vi "Demo_Main-Administrator-an.vi"() -> ()   [LabVIEW 2010]
uses:
  ControlCAN/ControlCAN.llb/DevType.ctl
  ControlCAN/ControlCAN.llb/CAN Channel.ctl
  ControlCAN/ControlCAN.llb/InitFlag.ctl
  ControlCAN/ControlCAN.llb/Mode.ctl
  ControlCAN/ControlCAN.llb/Fliter.ctl
  ControlCAN/ControlCAN.llb/VCI_CAN_OBJ.ctl
  ControlCAN/ControlCAN.llb/VCI_INIT_CONFIG.ctl
  ControlCAN/ControlCAN.llb/Return Val.ctl
  ControlCAN/ControlCAN.lvlib
panel:
  out "电流限制_回":dbl
  in  "电流限制_R":bool
  in  "电流限制_W":bool
  in  "电流限制":dbl
  in  "速度限制_R":bool
  in  "速度限制":dbl
  out "速度限制_回":dbl
  in  "速度限制_W":bool
  out "编码器线数_回":u16
  in  "编码器线数_R":bool
  in  "编码器线数_W":bool
  in  "编码器线数":u16
  in  "极对数_R":bool
  in  "极对数":u8
  out "极对数_回":u8
  in  "极对数_W":bool
  in  "电机自动校准":string(combo)="0"
  in  "电机校准_W":bool
  in  "对准角_R":bool
  in  "对准角":dbl format="%#.6f"
  out "对准角_回":dbl format="%#.6f"
  in  "对准角_W":bool
  in  "减速度_R":bool
  in  "减速度":dbl format="%#.6f"
  out "减速度_回":dbl format="%#.6f"
  in  "减速度_W":bool
  out "版本号":dbl format="%_3f"
  in  "看门狗周期_R":bool
  in  "看门狗周期":u16
  out "看门狗周期_回":u16
  in  "看门狗周期_W":bool
  in  "看门狗_W":bool
  in  "看门狗":string(combo)="开启"
  in  "监测周期_R":bool
  in  "监测周期":u16
  out "监测周期_回":u16
  in  "监测周期_W":bool
  out "ERRO7":bool
  out "ERRO6":bool
  out "ERRO5":bool
  out "ERRO4":bool
  out "ERRO3":bool
  out "高温":bool
  out "高压":bool
  out "低压":bool
  out "warn7":bool
  out "warn6":bool
  out "warn5":bool
  out "warn4":bool
  out "warn3":bool
  out "高温":bool
  out "warn1":bool
  out "warn0":bool
  out "温度":dbl format="%#.6f"
  out "转速":dbl(graph)
  out "CAN ID":u8 format="%x"
  out "数组":u8[](array[numeric]) format="%x"
  in  "DATA_SAVE_W":bool
  out "CI_K0_回":u16
  out "BI_K0_回":u16
  in  "CI_K0_R":bool
  in  "BI_K0_R":bool
  in  "CI_K0_W":bool
  in  "BI_K0_W":bool
  in  "C电流零偏":u16
  in  "B电流零偏":u16
  in  "AI_K0_R":bool
  in  "A电流零偏":u16
  out "AI_K0_回":u16
  in  "AI_K0_W":bool
  out "Sin":i32
  out "Cosin":i32
  in  "加速度_R":bool
  in  "加速度":dbl format="%#.6f"
  out "加速度_回":dbl format="%#.6f"
  in  "加速度_W":bool
  in  "速度环KI_R":bool
  in  "速度环KP_R":bool
  in  "速度环KI":dbl format="%#.6f"
  out "速度环KI_回":dbl format="%#.6f"
  in  "速度环KI_W":bool
  in  "速度环KP":dbl format="%#.6f"
  out "速度环KP_回":dbl format="%#.6f"
  in  "速度环KP_W":bool
  in  "电流环KI_R":bool
  in  "电流环KP_R":bool
  in  "电流环KI":dbl format="%#.6f"
  out "电流环KI_回":dbl format="%#.6f"
  in  "电流环KI_W":bool
  in  "电流环KP":dbl format="%#.6f"
  out "电流环KP_回":dbl format="%#.6f"
  in  "电流环KP_W":bool
  out "波形图表3":dbl(graph)
  out "波形图表2":dbl(graph)
  out "波形图表1":dbl(graph)
  out "sCnt":u32 caption="处理统计"
  out "模式_回":string(combo)="00"
  in  "模式_R":bool
  in  "设定电流_R":bool
  in  "设定位置_R":bool
  in  "设定速度_R":bool
  in  "存储路径":path
  in  "保存":bool
  out "保存_S":bool
  in  "模式_W":bool
  in  "模式":string(combo)="00"
  in  "设定电流":dbl format="%#.6f"
  out "设定电流_回":dbl format="%#.6f"
  in  "设定电流_W":bool
  in  "设定位置":dbl format="%#.6f"
  out "设定位置_回":dbl format="%#.6f"
  in  "设定位置_W":bool
  in  "设定速度":dbl format="%#.1f"
  out "设定速度_回":dbl format="%#.6f"
  in  "设定速度_W":bool
  in  "监测_W":bool
  in  "监测":string(combo)="30"
  out "电机ID_R":u32
  in  "Clear":bool
  out "Ualfa":dbl format="%#.6f"
  out "Ubate":dbl format="%#.6f"
  out "Uq":dbl format="%#.6f"
  out "Ud":dbl format="%#.6f"
  out "PWM1":u16
  out "PWM2":u16
  out "PWM3":u16
  out "sector":u8
  out "Iqnow":dbl
  out "Idnow":dbl
  out "Ialfa":dbl
  out "Ibeta":dbl
  out "A电流":dbl
  out "C电流":dbl
  out "B电流":dbl
  out "供电电压":dbl
  out "机械角度":dbl format="%.2f"
  out "电气角度":dbl
  out "转速":dbl
  out "CAN STD_ID":u32 format="%x"
  in  "电机ID":string(combo)="00"
  in  "电机ID_W":bool
  out "RecvCnt":u32 caption="接收统计"
  out "SendCnt":u32 caption="发送统计"
  in  "Format":u8(ring) items=["标准帧", "扩展帧"]
  in  "Type":u8(ring) items=["数据帧", "远程帧"]
  in  "Data":string="00 01 02 03 04 05 06 07"
  in  "ID":u32=291 format="0x%x"
  in  "Send":bool
  in  "RcvEnable":bool=TRUE
  out "Open":bool
  in  "Fliter":T1=1 items=["接收所有类型"=1, "只接收标准帧"=2, "只接收扩展帧"=3]
  in  "kBaudRate":u8(ring)=12 caption="波特率" items=["5k bps"=1, "10k bps"=2, "20k bps"=3, "40k bps"=4, "50k bps"=5, "80k bps"=6, "100k bps"=7, "125k bps"=8, "200k bps"=9, "250k bps"=10, "400k bps"=11, "500k bps"=12, "666k bps"=13, "800k bps"=14, "1000k bps"=15, "33.33k bps"=16, "66.66k bps"=17, "83.33k bps"=18]
  in  "Mode":T2 caption="工作模式" items=["正常工作", "仅侦听模式", "自测模式（环回）"]
  in  "InitFlag":T3 caption="初始化参数" items=["使用Flash参数", "使用界面设置参数"]
  in  "AccMask":u32=4294967295 caption="接收屏蔽码" format="%08x"
  in  "AccCode":u32 caption="接收过滤码" format="%08x"
  in  "Close":bool
  in  "Open":bool
  in  "Channel":T4 caption="CAN通道" items=["通道1", "通道2"]
  in  "DevType":T5=3 caption="设备类型" items=["USB-CAN"=2, "USB-CAN2"=3]
  # "发送指令帧包"
  # "CAN\n  ID"
  # "DATA"
  # "DATA"
  # "DATA"
  # "0"
  # "1"
  # "7"
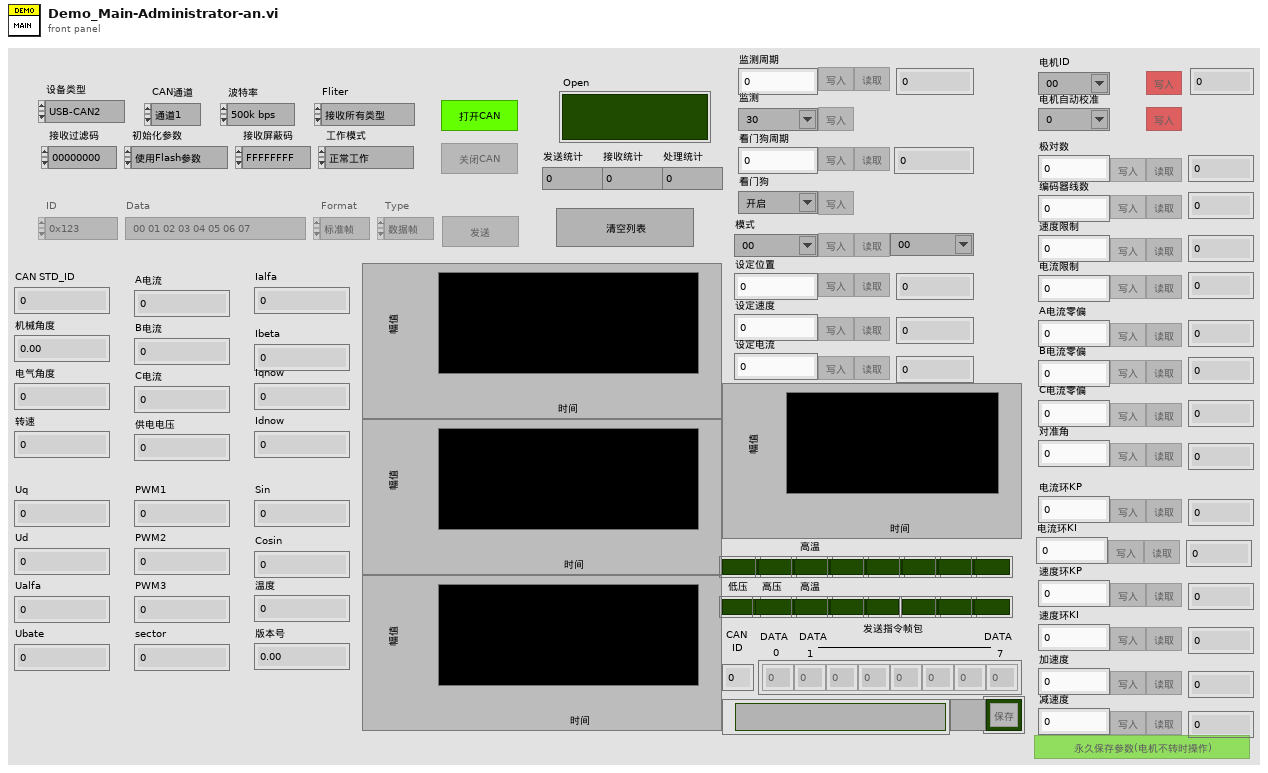
[diagram p1: front panel]
types:
  T1 = typedef "ControlCAN.lvlib/Fliter.ctl" = u8
  T2 = typedef "ControlCAN.lvlib/Mode.ctl" = u8
  T3 = typedef "ControlCAN.lvlib/InitFlag.ctl" = u32
  T4 = typedef "ControlCAN.lvlib/CAN Channel.ctl" = u32
  T5 = typedef "ControlCAN.lvlib/DevType.ctl" = u32
  T6 = typedef "ControlCAN.lvlib/VCI_CAN_OBJ.ctl" = cluster{"ID":u32, "TimeStamp":u32, "TimeFlag":u8, "SendType":u8, "RemoteFlag":u8, "ExternFlag":u8, "DataLen":u8, "Data":u8[], "Reserved":u8[]}
  T7 = cluster{"Type":enum16{"接收", "发送"}, "Channel":T4, "Time":timestamp, "VCI_CAN_OBJ":T6}[]
  T8 = typedef "ControlCAN.lvlib/VCI_INIT_CONFIG.ctl" = cluster{"AccCode":u32, "AccMask":u32, "InitFlag":T3, "Fliter":T1, "Timing0":u8, "Timing1":u8, "Mode":T2}
  T9 = cluster{"DevType":T5, "DevIndex":u32, "CanIndex":T4, "VCI_INIT_CONFIG":T8}
  T10 = typedef "ControlCAN.lvlib/Return Val.ctl" = i32
  T11 = enum16{"open", "replace", "create", "open or create", "replace or create", "replace or create with confirmation"}
  T12 = cluster{"[0]":cluster{"Type":enum16{"接收", "发送"}, "Channel":T4, "Time":timestamp, "VCI_CAN_OBJ":T6}}
  T13 = cluster{"Type":enum16{"接收", "发送"}, "Channel":T4, "Time":timestamp, "VCI_CAN_OBJ":T6}
  T14 = cluster{"Data[0]":u8, "Data[1]":u8, "Data[2]":u8, "Data[3]":u8, "Data[4]":u8, "Data[5]":u8, "Data[6]":u8, "Data[7]":u8}
  T15 = cluster{"Boolean array[0]":bool, "Boolean array[1]":bool, "Boolean array[2]":bool, "Boolean array[3]":bool, "Boolean array[4]":bool, "Boolean array[5]":bool, "Boolean array[6]":bool, "Boolean array[7]":bool}
  T16 = enum32{"invalid app kind", "Development System", "Run Time System", "Student Edition", "Embedded LabVIEW", "Evaluation", "Custom"}
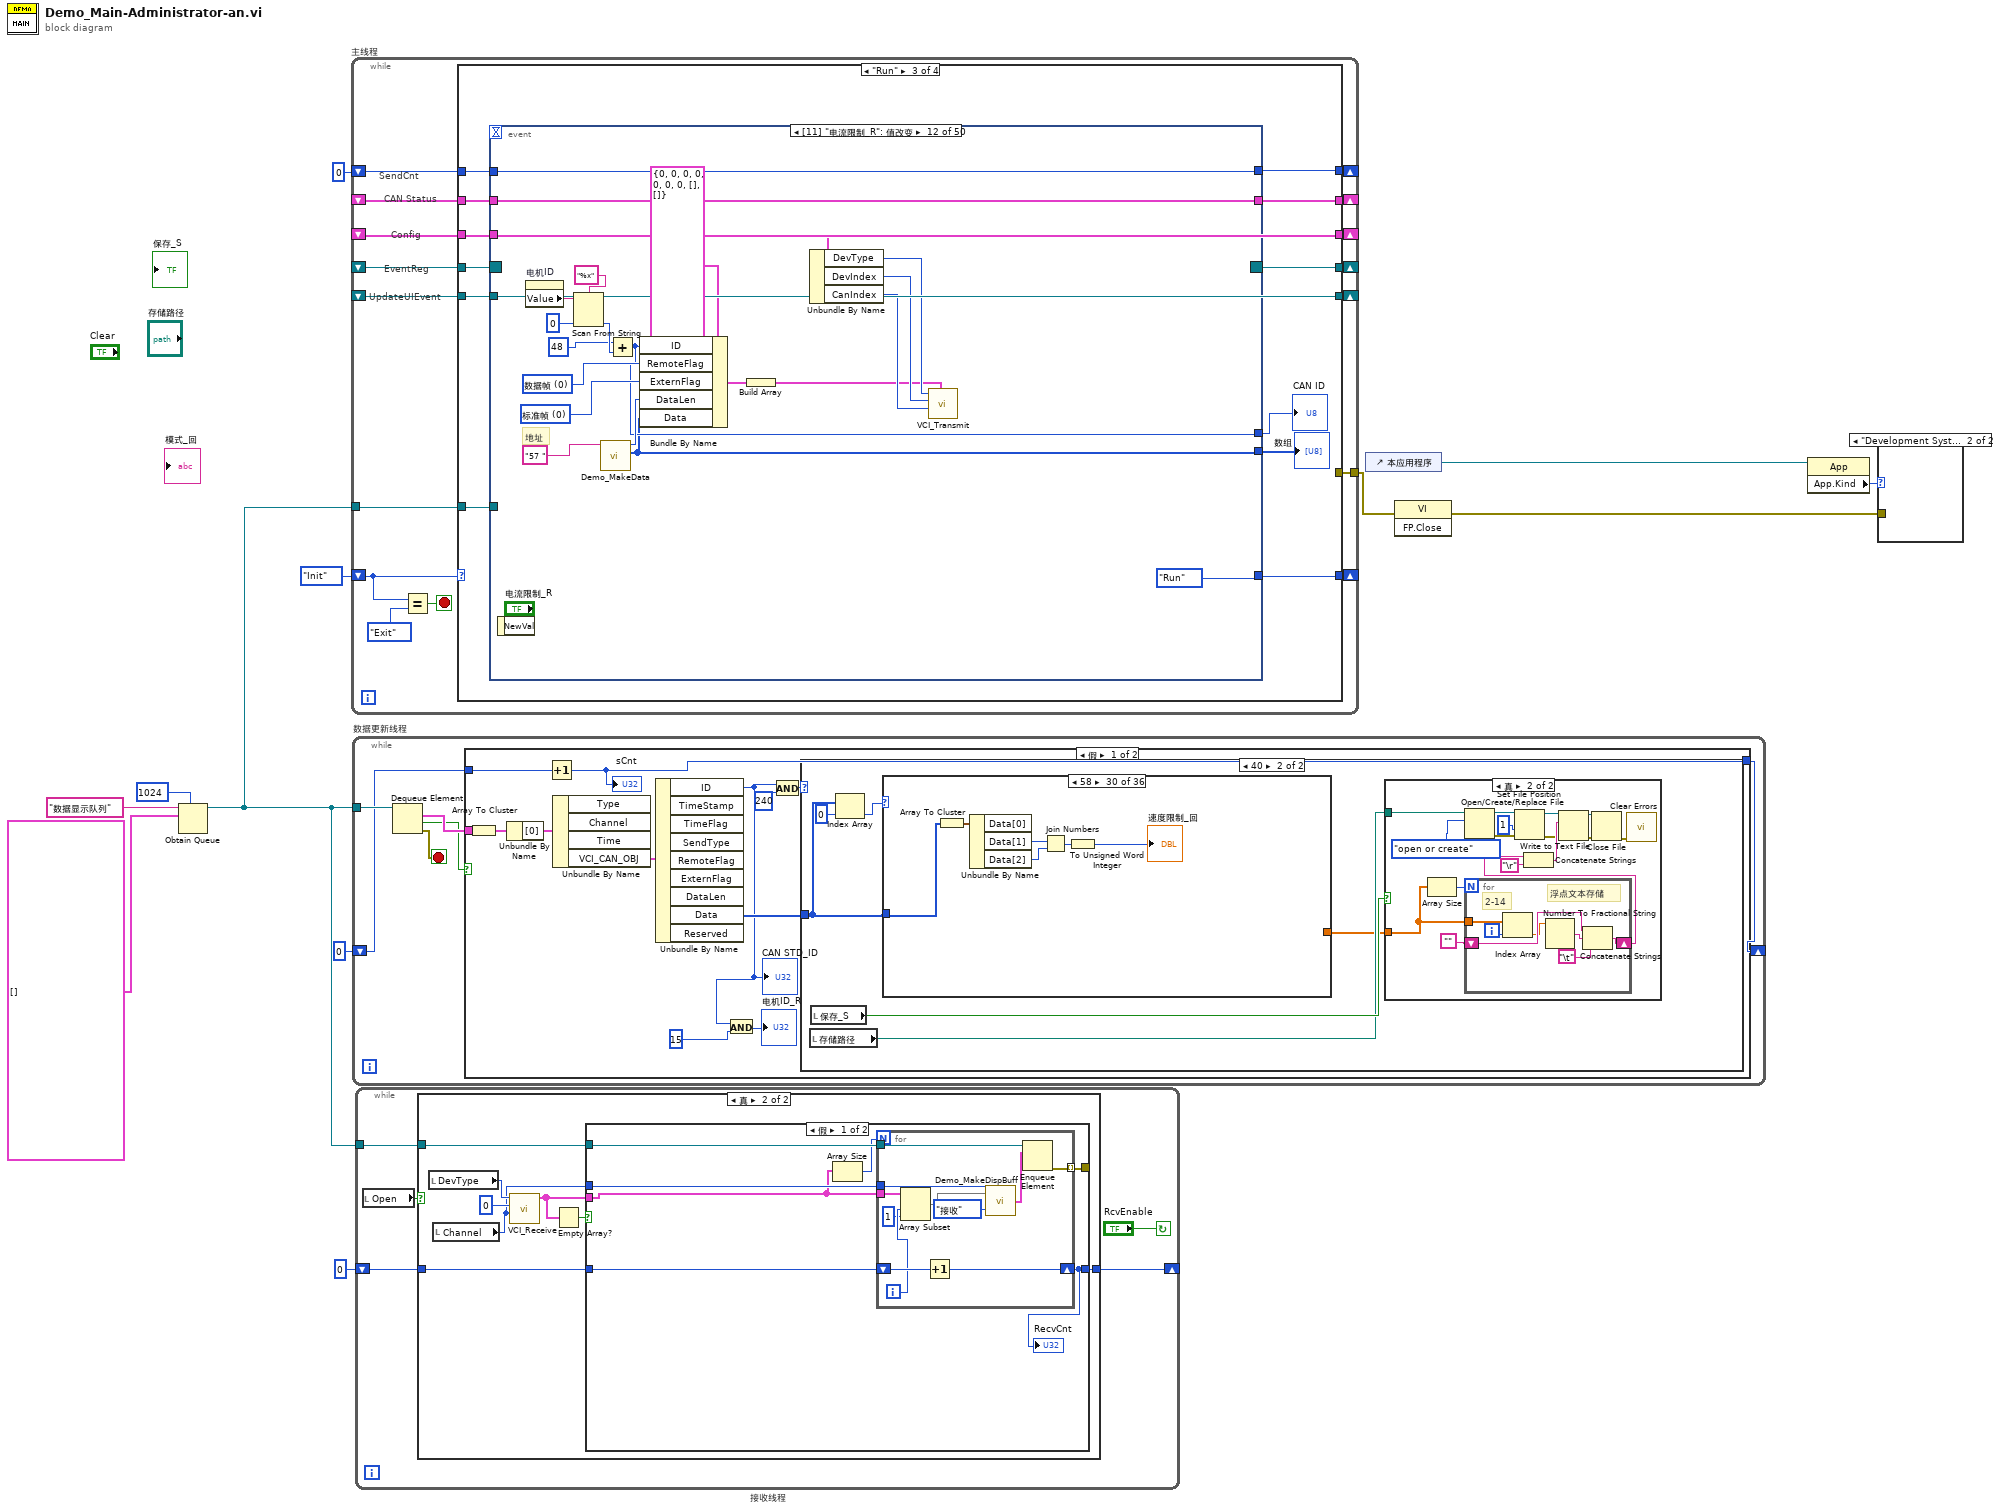
[diagram p0: block diagram]
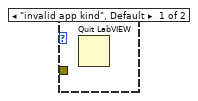
[diagram p2: hidden frame]
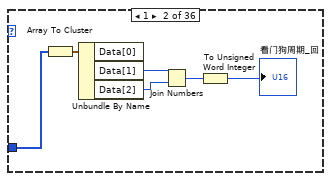
[diagram p6: hidden frame]
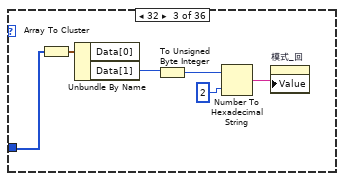
[diagram p7: hidden frame]
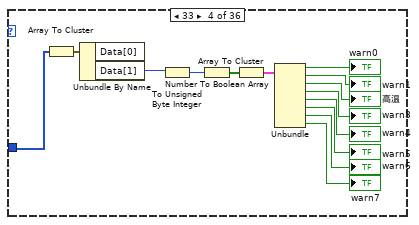
[diagram p8: hidden frame]
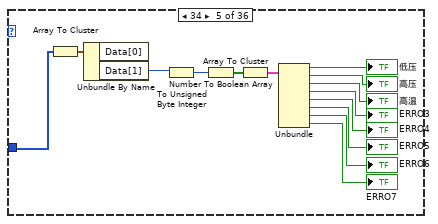
[diagram p9: hidden frame]
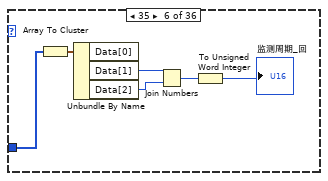
[diagram p10: hidden frame]
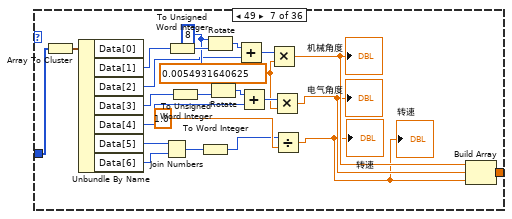
[diagram p11: hidden frame]
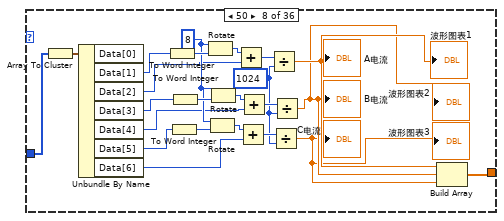
[diagram p12: hidden frame]
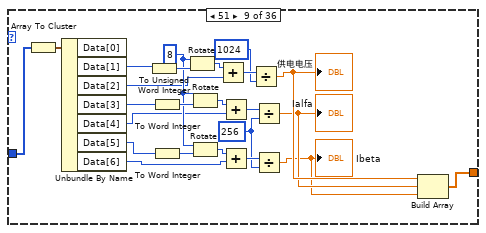
[diagram p13: hidden frame]
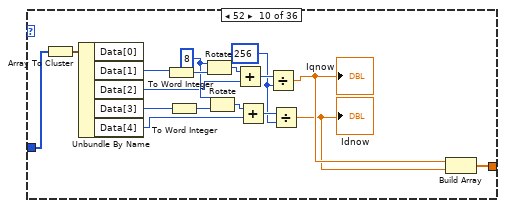
[diagram p14: hidden frame]
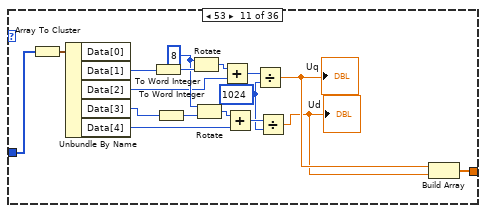
[diagram p15: hidden frame]
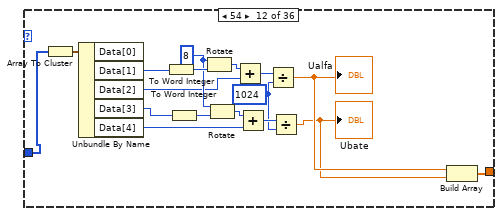
[diagram p16: hidden frame]
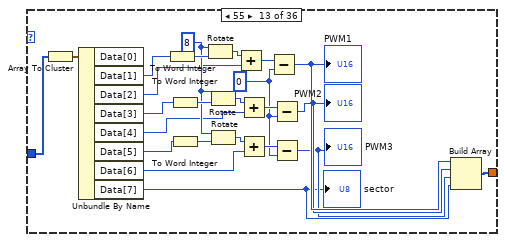
[diagram p17: hidden frame]
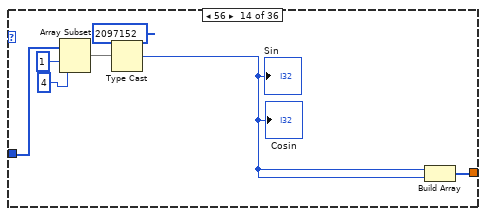
[diagram p18: hidden frame]
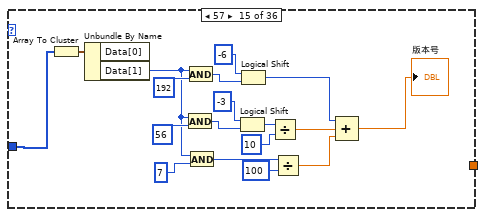
[diagram p19: hidden frame]
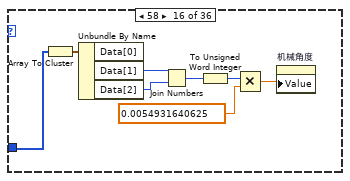
[diagram p20: hidden frame]
diagram:
  n1 = Obtain Queue(max queue size (-1, unlimited)=1024, name (unnamed)="数据显示队列" ("名称（未命名）"), element data type=T7 []) -> (queue out=w9:refnum<queue>)  [unwired: 2 in, 2 out]
  n2 = while "主线程" {
    shift-right: [w24] -> _
    shift-left: enum16{"Init", "Wait", "Run", "Exit"}."Init" -> [w27]
    shift-right: [w25] -> _
    shift-left: _ -> [w26]
    shift-right: [w23] -> _
    shift-left: _ -> [w22]
    tunnel: w9 -> [w21]
    shift-right: [w19] -> _
    shift-left: _ -> [w18]
    shift-right: [w17] -> _
    shift-left: _ -> [w16]
    shift-right: [w14] -> _
    shift-left: u32 0 -> [w15]
    tunnel: [w13] -> w4
    stop <- w28 stop-if-true
    # "CAN Status"
    # "Config"
    # "EventReg"
    # "UpdateUIEvent"
    # "SendCnt"
    n3 = Equal?(x=w27, y=enum16{"Init", "Wait", "Run", "Exit"}."Exit") -> (x = y?=w28:bool)
    n4 = case shown="\"Run\"" w27 {
      tunnel: w26 -> [_ w57 w158 w1270]
      tunnel: [w48 w56 w157 w1270] -> w25
      tunnel: [enum16{"Init", "Wait", "Run", "Exit"}."Wait" w53 w160 enum16{"Init", "Wait", "Run", "Exit"}."Exit"] -> w24
      tunnel: [w44 w54 w156 w1268] -> w23
      tunnel: w22 -> [_ w55 w156 w1268]
      tunnel: w21 -> [_ w52 w159 w1274]
      tunnel: [w36 w51 w154 w1273] -> w19
      tunnel: w18 -> [_ w51 w155 w1273]
      tunnel: [w35 w50 w153 w1271] -> w17
      tunnel: w16 -> [_ w50 w153 w1271]
      tunnel: w15 -> [w33 w49 w152 w1266]
      tunnel: [w33 w49 w151 w1266] -> w14
      tunnel: [_ _ _ errorcluster {"status"=FALSE, "code"=0, "source"=""} ("error constant")] -> w13
      frame "Init", Default {
        w37 = cluster{"CANOpen":bool} {"CANOpen"=FALSE}  # UpdateUI
        w47 = T9 {"DevType"=2, "DevIndex"=0, "CanIndex"=0, "VCI_INIT_CONFIG"={"AccCode"=0, "AccMask"=0, "InitFlag"=0, "Fliter"=0, "Timing0"=0, "Timing1"=0, "Mode"=0}}  # Config
        w48 = cluster{"Open":bool, "SendCnt":u32} {"Open"=FALSE, "SendCnt"=0}  # CAN Status
        n5 = property class="VI"("Front Panel.Closeable"=TRUE ("前面板窗口:可关闭")) -> ()  [unwired: 2 in, 2 out]
        n6 = invoke class="VI" method="Default Vals.Reinit All"() -> ()  [unwired: 3 in, 3 out]
        n7 = call "Demo_GetT0T1.vi"("kBaudRate"="kBaudRate") -> ("Timing0"=w30:u8, "Timing1"=w29:u8)
        n8 = Bundle By Name(cluster=w47, "DevType"="DevType", "CanIndex"="Channel", "VCI_INIT_CONFIG.AccCode"="AccCode", "VCI_INIT_CONFIG.AccMask"="AccMask", "VCI_INIT_CONFIG.InitFlag"="InitFlag", "VCI_INIT_CONFIG.Fliter"="Fliter", "VCI_INIT_CONFIG.Timing0"=w30, "VCI_INIT_CONFIG.Timing1"=w29, "VCI_INIT_CONFIG.Mode"="Mode") -> (w44:T9)
        n9 = local write "RcvEnable"(TRUE ("RcvEnable")) -> ()
        n10 = Create User Event(user event datatype=w37) -> (user event=w35:refnum<user-event>)  [unwired: 1 in, 1 out]
        n11 = register-events(w35) -> (reference out=w36:refnum<event-registration>)  [unwired: 2 in, 1 out]
      }
      frame "Wait" {
        n12 = event shown="[1] 前面板关闭？" {
          selector: _ -> [_ _ _ _ _ _ _ _ _ _]
          dyn-events: _ -> [_ _ _ _ _ _ _ _ _ _]
          timeout: _ -> [_ _ _ _ _ _ _ _ _ _]
          tunnel: w57 -> [w61 w101 w111 w116 w121 w126 w131 w136 w143 w148]
          tunnel: [w60 w101 w111 w116 w121 w126 w131 w136 w143 w148] -> w56
          tunnel: w55 -> [w71 w100 w110 w115 w120 w125 w130 w135 w142 w147]
          tunnel: [w71 w100 w109 w113 w118 w123 w128 w133 w141 w145] -> w54
          tunnel: [w62 enum16{"Init", "Wait", "Run", "Exit"}."Exit" enum16{"Init", "Wait", "Run", "Exit"}."Wait" enum16{"Init", "Wait", "Run", "Exit"}."Wait" enum16{"Init", "Wait", "Run", "Exit"}."Wait" enum16{"Init", "Wait", "Run", "Exit"}."Wait" enum16{"Init", "Wait", "Run", "Exit"}."Wait" enum16{"Init", "Wait", "Run", "Exit"}."Wait" enum16{"Init", "Wait", "Run", "Exit"}."Wait" enum16{"Init", "Wait", "Run", "Exit"}."Wait"] -> w53
          tunnel: w52 -> [_ _ _ _ _ _ _ _ _ _]
          tunnel: w50 -> [w59 _ _ _ _ _ _ _ _ _]
          event "Open": Value Change {
            w65 = T10 1 items=["OK"=1, "ERROR1"=0, "ERROR2"=-1] ("y")
            # "打开CAN的步骤：\n1.Open\n2.Init\n3.Start"
            n13 = event-data() -> ()  [unwired: 2 out]
            n14 = Unbundle By Name(w71) -> ("DevType"=w70:T5, "DevIndex"=w69:u32)
            n15 = call "VCI_OpenDevice.vi"("DevIndex"=w69, "DevType"=w70) -> ("error out"=w66:errorcluster, "Return Val"=w68:T10)  [unwired: 2 in, 6 out]
            n16 = Equal?(x=w68, y=w65) -> (x = y?=w67:bool)
            n17 = case shown="真" w67 {
              tunnel: w66 -> [_ w86]
              tunnel: w71 -> [_ w85]
              tunnel: w65 -> [_ w77]
              tunnel: [_ w76] -> w58
              frame False {
              }
              frame True {
                n18 = Unbundle By Name(w85) -> ("VCI_INIT_CONFIG"=w84:T8, "DevType"=w80:T5, "DevIndex"=w79:u32, "CanIndex"=w78:T4)
                n19 = call "VCI_InitCAN.vi"("VCI_INIT_CONFIG"=w84, "error in (no error)"=w86, "CANIndex"=w78, "DevIndex"=w79, "DevType"=w80) -> ("error out"=w81:errorcluster, "Return Val"=w83:T10)  [unwired: 5 out]
                n20 = Equal?(x=w77, y=w83) -> (x = y?=w82:bool)
                n21 = case shown="真" w82 {
                  tunnel: w81 -> [_ w97]
                  tunnel: w80 -> [_ w96]
                  tunnel: w79 -> [_ w95]
                  tunnel: w78 -> [_ w94]
                  tunnel: w77 -> [_ w92]
                  tunnel: [_ w88] -> w76
                  frame False {
                  }
                  frame True {
                    n22 = call "VCI_StartCAN.vi"("error in (no error)"=w97, "CANIndex"=w94, "DevIndex"=w95, "DevType"=w96) -> ("error out"=w90:errorcluster, "Return Val"=w93:T10)  [unwired: 6 out]
                    n23 = Unbundle By Name(w90) -> ("status"=w87:bool)
                    n24 = Equal?(x=w92, y=w93) -> (x = y?=w91:bool)
                    n25 = Not(x=w87) -> (.not. x?=w89:bool)
                    n26 = And(x=w91, y=w89) -> (x .and. y?=w88:bool)
                  }
                }
              }
            }
            n27 = case shown="真" w58 {
              tunnel: w59 -> [_ w75]
              tunnel: w58 -> [_ w73]
              frame False {
              }
              frame True {
                n28 = Bundle By Name(cluster=cluster{"CANOpen":bool} {"CANOpen"=FALSE} ("事件数据"), "CANOpen"=w73) -> (w72:cluster{"CANOpen":bool})
                n29 = Generate User Event(user event=w75, event data cluster=w72) -> ()  [unwired: 1 in, 2 out]
              }
            }
            n30 = Select(t=enum16{"Init", "Wait", "Run", "Exit"}."Run", s=w58, f=enum16{"Init", "Wait", "Run", "Exit"}."Wait") -> (s? t:f=w62:enum16{"Init", "Wait", "Run", "Exit"})
            n31 = Bundle By Name(cluster=w61, "Open"=w58) -> (w60:cluster{"Open":bool, "SendCnt":u32})
          }
          event Panel Close? {
            n32 = event-data() -> ()  [unwired: 2 out]
            n33 = event-data("Discard?"=TRUE ("放弃？")) -> ()  [unwired: 1 in, 1 out]
          }
          event Value Change {
            w107 = T5 3 items=["USB-CAN"=2, "USB-CAN2"=3] ("y")
            n34 = event-data() -> ("NewVal"=w108:T5)  [unwired: 1 out]
            n35 = Equal?(x=w108, y=w107) -> (x = y?=w106:bool)
            n36 = Bundle By Name(cluster=w110, "DevType"=w108) -> (w109:T9)
            n37 = Select(t=i32[] [] ("禁用项[]"), s=w106, f=i32[] [1] ("禁用项[]")) -> (s? t:f=w105:i32[])
            n38 = property on="Channel" class="Ring (严格)"("Disabled Items []"=w105) -> ()  [unwired: 2 in, 2 out]
          }
          event Value Change {
            n39 = event-data() -> ("NewVal"=w114:T4)  [unwired: 1 out]
            n40 = Bundle By Name(cluster=w115, "CanIndex"=w114) -> (w113:T9)
          }
          event "AccCode": Value Change {
            n41 = event-data() -> ("NewVal"=w119:u32)  [unwired: 1 out]
            n42 = Bundle By Name(cluster=w120, "VCI_INIT_CONFIG.AccCode"=w119) -> (w118:T9)
          }
          event "AccMask": Value Change {
            n43 = event-data() -> ("NewVal"=w124:u32)  [unwired: 1 out]
            n44 = Bundle By Name(cluster=w125, "VCI_INIT_CONFIG.AccMask"=w124) -> (w123:T9)
          }
          event Value Change {
            n45 = event-data() -> ("NewVal"=w129:T3)  [unwired: 1 out]
            n46 = Bundle By Name(cluster=w130, "VCI_INIT_CONFIG.InitFlag"=w129) -> (w128:T9)
          }
          event Value Change {
            n47 = event-data() -> ("NewVal"=w134:T2)  [unwired: 1 out]
            n48 = Bundle By Name(cluster=w135, "VCI_INIT_CONFIG.Mode"=w134) -> (w133:T9)
          }
          event "kBaudRate": Value Change {
            n49 = event-data() -> ("NewVal"=w139:u8)  [unwired: 1 out]
            n50 = call "Demo_GetT0T1.vi"("kBaudRate"=w139) -> ("Timing0"=w138:u8, "Timing1"=w137:u8)
            n51 = Bundle By Name(cluster=w142, "VCI_INIT_CONFIG.Timing0"=w138, "VCI_INIT_CONFIG.Timing1"=w137) -> (w141:T9)
          }
          event Value Change {
            n52 = event-data() -> ("NewVal"=w146:T1)  [unwired: 1 out]
            n53 = Bundle By Name(cluster=w147, "VCI_INIT_CONFIG.Fliter"=w146) -> (w145:T9)
          }
        }
      }
      frame "Run" {
        n54 = event shown="[11] \"电流限制_R\": 值改变" {
          selector: w155 -> [_ _ _ _ _ _ _ _ _ _ _ _ _ _ _ _ _ _ _ _ _ _ _ _ _ _ _ _ _ _ _ _ _ _ _ _ _ _ _ _ _ _ _ _ _ _ _ _ _ _]
          dyn-events: [_ _ _ _ _ _ _ _ _ _ _ _ _ _ _ _ _ _ _ _ _ _ _ _ _ _ _ _ _ _ _ _ _ _ _ _ _ _ _ _ _ _ _ _ _ _ _ _ _ _] -> w154
          timeout: _ -> [_ _ _ _ _ _ _ _ _ _ _ _ _ _ _ _ _ _ _ _ _ _ _ _ _ _ _ _ _ _ _ _ _ _ _ _ _ _ _ _ _ _ _ _ _ _ _ _ _ _]
          tunnel: [enum16{"Init", "Wait", "Run", "Exit"}."Run" enum16{"Init", "Wait", "Run", "Exit"}."Run" enum16{"Init", "Wait", "Run", "Exit"}."Run" enum16{"Init", "Wait", "Run", "Exit"}."Run" enum16{"Init", "Wait", "Run", "Exit"}."Run" enum16{"Init", "Wait", "Run", "Exit"}."Run" enum16{"Init", "Wait", "Run", "Exit"}."Run" enum16{"Init", "Wait", "Run", "Exit"}."Run" enum16{"Init", "Wait", "Run", "Exit"}."Run" enum16{"Init", "Wait", "Run", "Exit"}."Run" enum16{"Init", "Wait", "Run", "Exit"}."Run" enum16{"Init", "Wait", "Run", "Exit"}."Run" enum16{"Init", "Wait", "Run", "Exit"}."Run" enum16{"Init", "Wait", "Run", "Exit"}."Run" enum16{"Init", "Wait", "Run", "Exit"}."Run" enum16{"Init", "Wait", "Run", "Exit"}."Run" enum16{"Init", "Wait", "Run", "Exit"}."Run" enum16{"Init", "Wait", "Run", "Exit"}."Run" enum16{"Init", "Wait", "Run", "Exit"}."Run" enum16{"Init", "Wait", "Run", "Exit"}."Run" enum16{"Init", "Wait", "Run", "Exit"}."Run" enum16{"Init", "Wait", "Run", "Exit"}."Run" enum16{"Init", "Wait", "Run", "Exit"}."Run" enum16{"Init", "Wait", "Run", "Exit"}."Run" enum16{"Init", "Wait", "Run", "Exit"}."Run" enum16{"Init", "Wait", "Run", "Exit"}."Run" enum16{"Init", "Wait", "Run", "Exit"}."Run" enum16{"Init", "Wait", "Run", "Exit"}."Run" enum16{"Init", "Wait", "Run", "Exit"}."Run" enum16{"Init", "Wait", "Run", "Exit"}."Run" enum16{"Init", "Wait", "Run", "Exit"}."Run" enum16{"Init", "Wait", "Run", "Exit"}."Run" enum16{"Init", "Wait", "Run", "Exit"}."Run" enum16{"Init", "Wait", "Run", "Exit"}."Run" enum16{"Init", "Wait", "Run", "Exit"}."Run" enum16{"Init", "Wait", "Run", "Exit"}."Run" enum16{"Init", "Wait", "Run", "Exit"}."Run" enum16{"Init", "Wait", "Run", "Exit"}."Run" enum16{"Init", "Wait", "Run", "Exit"}."Run" enum16{"Init", "Wait", "Run", "Exit"}."Run" enum16{"Init", "Wait", "Run", "Exit"}."Run" enum16{"Init", "Wait", "Run", "Exit"}."Run" enum16{"Init", "Wait", "Run", "Exit"}."Run" enum16{"Init", "Wait", "Run", "Exit"}."Run" enum16{"Init", "Wait", "Run", "Exit"}."Run" enum16{"Init", "Wait", "Run", "Exit"}."Run" enum16{"Init", "Wait", "Run", "Exit"}."Run" enum16{"Init", "Wait", "Run", "Exit"}."Run" enum16{"Init", "Wait", "Run", "Exit"}."Run" w1259] -> w160
          tunnel: w159 -> [_ _ _ _ _ _ _ _ _ _ _ _ _ _ _ _ _ _ _ _ _ _ _ _ _ _ _ _ _ _ _ _ _ _ _ _ _ _ _ _ _ _ _ _ _ _ _ _ _ _]
          tunnel: [w162 w179 w196 w219 w241 w262 w286 w307 w334 w355 w382 w403 w427 w448 w469 w488 w509 w525 w563 w584 w610 w636 w662 w688 w714 w740 w766 w792 w818 w842 w866 w890 w917 w938 w959 w980 w1001 w1022 w1043 w1064 w1085 w1106 w1127 w1148 w1169 w1190 w1211 w1239 w1245 w1264] -> w157
          tunnel: w158 -> [w162 w179 w196 w219 w241 w262 w286 w307 w334 w355 w382 w403 w427 w448 w469 w488 w509 w525 w563 w584 w610 w636 w662 w688 w714 w740 w766 w792 w818 w842 w866 w890 w917 w938 w959 w980 w1001 w1022 w1043 w1064 w1085 w1106 w1127 w1148 w1169 w1190 w1211 w1239 w1247 w1264]
          tunnel: w156 -> [_ w174 w186 w201 w224 w245 w267 w290 w315 w338 w360 w386 w408 w431 w458 w474 w492 w515 w545 w567 w595 w618 w644 w667 w693 w719 w745 w771 w797 w823 w847 w871 w898 w921 w942 w963 w984 w1005 w1026 w1047 w1068 w1089 w1110 w1131 w1152 w1173 w1194 _ w1252 _]
          tunnel: w153 -> [_ _ _ _ _ _ _ _ _ _ _ _ _ _ _ _ _ _ _ _ _ _ _ _ _ _ _ _ _ _ _ _ _ _ _ _ _ _ _ _ _ _ _ _ _ _ _ _ w1244 _]
          tunnel: w152 -> [w161 w167 w195 w218 w240 w261 w285 w306 w333 w354 w381 w402 w426 w447 w468 w487 w508 w524 w562 w583 w609 w635 w661 w687 w713 w739 w765 w791 w817 w841 w865 w889 w916 w937 w958 w979 w1000 w1021 w1042 w1063 w1084 w1105 w1126 w1147 w1168 w1189 w1210 w1238 w1240 w1258]
          tunnel: [w161 w166 w195 w218 w240 w261 w285 w306 w333 w354 w381 w402 w426 w447 w468 w487 w508 w524 w562 w583 w609 w635 w661 w687 w713 w739 w765 w791 w817 w841 w865 w889 w916 w937 w958 w979 w1000 w1021 w1042 w1063 w1084 w1105 w1126 w1147 w1168 w1189 w1210 w1238 w1240 w1258] -> w151
          tunnel: [_ _ w182 w199 w222 w243 w264 w288 w313 w336 w358 w384 w406 w429 w450 w472 w490 w511 w543 w565 w586 w612 w638 w664 w690 w716 w742 w768 w795 w820 w844 w868 w896 w919 w940 w961 w982 w1003 w1024 w1045 w1066 w1087 w1108 w1129 w1150 w1171 w1192 _ _ _] -> w150
          tunnel: [_ _ w181 w200 w223 w244 w265 w289 w314 w337 w359 w385 w407 w430 w449 w473 w491 w514 w542 w564 w585 w611 w637 w663 w689 w715 w741 w767 w794 w819 w843 w867 w897 w918 w939 w960 w981 w1002 w1023 w1044 w1065 w1086 w1109 w1128 w1149 w1170 w1193 _ _ _] -> w149
          event Timeout {
            n55 = event-data() -> ()  [unwired: 3 out]
          }
          event "Send": Value Change {
            n56 = event-data() -> ()  [unwired: 2 out]
            n57 = Increment(x=w167) -> (x+1=w166:u32)
            "SendCnt" <- w166
            n58 = call "Demo_MakeData.vi"("DataString"="Data") -> ("Data"=w169:u8[], "DataLen"=w170:u8)  [unwired: 9 out]
            n59 = Bundle By Name(cluster=T6 {"ID"=0, "TimeStamp"=0, "TimeFlag"=0, "SendType"=0, "RemoteFlag"=0, "ExternFlag"=0, "DataLen"=0, "Data"=[], "Reserved"=[]} ("Send"), "ID"="ID", "RemoteFlag"="Type", "ExternFlag"="Format", "DataLen"=w170, "Data"=w169) -> (w164:T6)
            n60 = Build Array(w164) -> (w165:T6[])
            n61 = Unbundle By Name(w174) -> ("DevType"=w173:T5, "DevIndex"=w172:u32, "CanIndex"=w168:T4)
            n62 = call "VCI_Transmit.vi"("Buffer"=w165, "CANIndex"=w168, "DevIndex"=w172, "DevType"=w173) -> ()  [unwired: 1 in, 7 out]
          }
          event "电机ID_W": Value Change {
            w185 = u8 0 items=["数据帧", "遥控帧"]
            w181 = u32 138
            w184 = u8 0 items=["标准帧", "扩展帧"]
            n63 = event-data() -> ()  [unwired: 2 out]
            n64 = call "Demo_MakeData.vi"("DataString"="电机ID") -> ("Data"=w182:u8[], "DataLen"=w190:u8)  [unwired: 9 out]
            n65 = Bundle By Name(cluster=T6 {"ID"=0, "TimeStamp"=0, "TimeFlag"=0, "SendType"=0, "RemoteFlag"=0, "ExternFlag"=0, "DataLen"=0, "Data"=[], "Reserved"=[]} ("Send"), "ID"=w181, "RemoteFlag"=w185, "ExternFlag"=w184, "DataLen"=w190, "Data"=w182) -> (w187:T6)
            n66 = Build Array(w187) -> (w188:T6[])
            n67 = Unbundle By Name(w186) -> ("DevType"=w192:T5, "DevIndex"=w191:u32, "CanIndex"=w189:T4)
            n68 = call "VCI_Transmit.vi"("Buffer"=w188, "CANIndex"=w189, "DevIndex"=w191, "DevType"=w192) -> ()  [unwired: 1 in, 7 out]
          }
          event "电机校准_W": Value Change {
            w216 = u8 0 items=["数据帧", "遥控帧"]
            w217 = u8 0 items=["标准帧", "扩展帧"]
            # "地址"
            n69 = event-data() -> ()  [unwired: 2 out]
            n70 = property on="电机ID" class="CmbBox"() -> ("Value"=w207:string)  [unwired: 2 in, 2 out]
            n71 = Concatenate Strings("20 ", "AA 01 02 03 04 05 55") -> (w203:string)
            n72 = Scan From String(format string="%x" ("格式字符串"), input string=w207, default 1=u8 0) -> (output 1=w204:u8)  [unwired: 2 in, 3 out]
            n73 = call "Demo_MakeData.vi"("DataString"=w203) -> ("Data"=w199:u8[], "DataLen"=w212:u8)  [unwired: 9 out]
            n74 = Add(x=u32 16, y=w204) -> (x+y=w200:u32)
            n75 = Bundle By Name(cluster=T6 {"ID"=0, "TimeStamp"=0, "TimeFlag"=0, "SendType"=0, "RemoteFlag"=0, "ExternFlag"=0, "DataLen"=0, "Data"=[], "Reserved"=[]} ("Send"), "ID"=w200, "RemoteFlag"=w216, "ExternFlag"=w217, "DataLen"=w212, "Data"=w199) -> (w215:T6)
            n76 = Build Array(w215) -> (w214:T6[])
            n77 = Unbundle By Name(w201) -> ("DevType"=w210:T5, "DevIndex"=w211:u32, "CanIndex"=w213:T4)
            n78 = call "VCI_Transmit.vi"("Buffer"=w214, "CANIndex"=w213, "DevIndex"=w211, "DevType"=w210) -> ()  [unwired: 1 in, 7 out]
          }
          event "极对数_W": Value Change {
            w236 = u8 0 items=["数据帧", "遥控帧"]
            w237 = u8 0 items=["标准帧", "扩展帧"]
            # "索引地址"
            n79 = event-data() -> ()  [unwired: 2 out]
            n80 = property on="电机ID" class="CmbBox"() -> ("Value"=w228:string)  [unwired: 2 in, 2 out]
            n81 = Scan From String(format string="%x" ("格式字符串"), input string=w228, default 1=u8 0) -> (output 1=w225:u8)  [unwired: 2 in, 3 out]
            n82 = Add(x=u32 16, y=w225) -> (x+y=w223:u32)
            n83 = Build Array(u8 94, "极对数") -> (w222:u8[])
            n84 = Bundle By Name(cluster=T6 {"ID"=0, "TimeStamp"=0, "TimeFlag"=0, "SendType"=0, "RemoteFlag"=0, "ExternFlag"=0, "DataLen"=0, "Data"=[], "Reserved"=[]} ("Send"), "ID"=w223, "RemoteFlag"=w236, "ExternFlag"=w237, "DataLen"=u8 2, "Data"=w222) -> (w235:T6)
            n85 = Build Array(w235) -> (w234:T6[])
            n86 = Unbundle By Name(w224) -> ("DevType"=w231:T5, "DevIndex"=w232:u32, "CanIndex"=w233:T4)
            n87 = call "VCI_Transmit.vi"("Buffer"=w234, "CANIndex"=w233, "DevIndex"=w232, "DevType"=w231) -> ()  [unwired: 1 in, 7 out]
          }
          event "极对数_R": Value Change {
            w248 = u8 0 items=["数据帧", "遥控帧"]
            w247 = u8 0 items=["标准帧", "扩展帧"]
            # "地址"
            n88 = event-data() -> ()  [unwired: 2 out]
            n89 = property on="电机ID" class="CmbBox"() -> ("Value"=w257:string)  [unwired: 2 in, 2 out]
            n90 = Scan From String(format string="%x" ("格式字符串"), input string=w257, default 1=u8 0) -> (output 1=w260:u8)  [unwired: 2 in, 3 out]
            n91 = call "Demo_MakeData.vi"("DataString"="5E") -> ("Data"=w243:u8[], "DataLen"=w252:u8)  [unwired: 9 out]
            n92 = Add(x=u32 48, y=w260) -> (x+y=w244:u32)
            n93 = Bundle By Name(cluster=T6 {"ID"=0, "TimeStamp"=0, "TimeFlag"=0, "SendType"=0, "RemoteFlag"=0, "ExternFlag"=0, "DataLen"=0, "Data"=[], "Reserved"=[]} ("Send"), "ID"=w244, "RemoteFlag"=w248, "ExternFlag"=w247, "DataLen"=w252, "Data"=w243) -> (w249:T6)
            n94 = Build Array(w249) -> (w250:T6[])
            n95 = Unbundle By Name(w245) -> ("DevType"=w254:T5, "DevIndex"=w253:u32, "CanIndex"=w251:T4)
            n96 = call "VCI_Transmit.vi"("Buffer"=w250, "CANIndex"=w251, "DevIndex"=w253, "DevType"=w254) -> ()  [unwired: 1 in, 7 out]
          }
          event "编码器线数_W": Value Change {
            w279 = u8 0 items=["数据帧", "遥控帧"]
            w280 = u8 0 items=["标准帧", "扩展帧"]
            # "索引地址"
            n97 = event-data() -> ()  [unwired: 2 out]
            n98 = property on="电机ID" class="CmbBox"() -> ("Value"=w271:string)  [unwired: 2 in, 2 out]
            n99 = Scan From String(format string="%x" ("格式字符串"), input string=w271, default 1=u8 0) -> (output 1=w268:u8)  [unwired: 2 in, 3 out]
            n100 = Split Number(x="编码器线数") -> (hi(x)=w283:u8, lo(x)=w284:u8)
            n101 = Add(x=u32 16, y=w268) -> (x+y=w265:u32)
            n102 = Build Array(u8 95, w283, w284) -> (w264:u8[])
            n103 = Bundle By Name(cluster=T6 {"ID"=0, "TimeStamp"=0, "TimeFlag"=0, "SendType"=0, "RemoteFlag"=0, "ExternFlag"=0, "DataLen"=0, "Data"=[], "Reserved"=[]} ("Send"), "ID"=w265, "RemoteFlag"=w279, "ExternFlag"=w280, "DataLen"=u8 3, "Data"=w264) -> (w278:T6)
            n104 = Build Array(w278) -> (w277:T6[])
            n105 = Unbundle By Name(w267) -> ("DevType"=w274:T5, "DevIndex"=w275:u32, "CanIndex"=w276:T4)
            n106 = call "VCI_Transmit.vi"("Buffer"=w277, "CANIndex"=w276, "DevIndex"=w275, "DevType"=w274) -> ()  [unwired: 1 in, 7 out]
          }
          event "编码器线数_R": Value Change {
            w293 = u8 0 items=["数据帧", "遥控帧"]
            w292 = u8 0 items=["标准帧", "扩展帧"]
            # "地址"
            n107 = event-data() -> ()  [unwired: 2 out]
            n108 = property on="电机ID" class="CmbBox"() -> ("Value"=w302:string)  [unwired: 2 in, 2 out]
            n109 = Scan From String(format string="%x" ("格式字符串"), input string=w302, default 1=u8 0) -> (output 1=w305:u8)  [unwired: 2 in, 3 out]
            n110 = call "Demo_MakeData.vi"("DataString"="5F ") -> ("Data"=w288:u8[], "DataLen"=w297:u8)  [unwired: 9 out]
            n111 = Add(x=u32 48, y=w305) -> (x+y=w289:u32)
            n112 = Bundle By Name(cluster=T6 {"ID"=0, "TimeStamp"=0, "TimeFlag"=0, "SendType"=0, "RemoteFlag"=0, "ExternFlag"=0, "DataLen"=0, "Data"=[], "Reserved"=[]} ("Send"), "ID"=w289, "RemoteFlag"=w293, "ExternFlag"=w292, "DataLen"=w297, "Data"=w288) -> (w294:T6)
            n113 = Build Array(w294) -> (w295:T6[])
            n114 = Unbundle By Name(w290) -> ("DevType"=w299:T5, "DevIndex"=w298:u32, "CanIndex"=w296:T4)
            n115 = call "VCI_Transmit.vi"("Buffer"=w295, "CANIndex"=w296, "DevIndex"=w298, "DevType"=w299) -> ()  [unwired: 1 in, 7 out]
          }
          event "速度限制_W": Value Change {
            w319 = u8 0 items=["数据帧", "遥控帧"]
            w318 = u8 0 items=["标准帧", "扩展帧"]
            # "索引地址"
            n116 = event-data() -> ()  [unwired: 2 out]
            n117 = property on="电机ID" class="CmbBox"() -> ("Value"=w327:string)  [unwired: 2 in, 2 out]
            n118 = Multiply ("乘")(x="速度限制", y=i16 1) -> (x*y=w311:i16)
            n119 = Scan From String(format string="%x" ("格式字符串"), input string=w327, default 1=u8 0) -> (output 1=w330:u8)  [unwired: 2 in, 3 out]
            n120 = Absolute Value(x=w311) -> (abs(x)=w308:i16)
            n121 = Add(x=u32 16, y=w330) -> (x+y=w314:u32)
            n122 = Split Number(x=w308) -> (hi(x)=w331:u8, lo(x)=w332:u8)
            n123 = Build Array(u8 88, w331, w332) -> (w313:u8[])
            n124 = Bundle By Name(cluster=T6 {"ID"=0, "TimeStamp"=0, "TimeFlag"=0, "SendType"=0, "RemoteFlag"=0, "ExternFlag"=0, "DataLen"=0, "Data"=[], "Reserved"=[]} ("Send"), "ID"=w314, "RemoteFlag"=w319, "ExternFlag"=w318, "DataLen"=u8 3, "Data"=w313) -> (w320:T6)
            n125 = Build Array(w320) -> (w321:T6[])
            n126 = Unbundle By Name(w315) -> ("DevType"=w324:T5, "DevIndex"=w323:u32, "CanIndex"=w322:T4)
            n127 = call "VCI_Transmit.vi"("Buffer"=w321, "CANIndex"=w322, "DevIndex"=w323, "DevType"=w324) -> ()  [unwired: 1 in, 7 out]
          }
          event "速度限制_R": Value Change {
            w341 = u8 0 items=["数据帧", "遥控帧"]
            w340 = u8 0 items=["标准帧", "扩展帧"]
            # "地址"
            n128 = event-data() -> ()  [unwired: 2 out]
            n129 = property on="电机ID" class="CmbBox"() -> ("Value"=w350:string)  [unwired: 2 in, 2 out]
            n130 = Scan From String(format string="%x" ("格式字符串"), input string=w350, default 1=u8 0) -> (output 1=w353:u8)  [unwired: 2 in, 3 out]
            n131 = call "Demo_MakeData.vi"("DataString"="58") -> ("Data"=w336:u8[], "DataLen"=w345:u8)  [unwired: 9 out]
            n132 = Add(x=u32 48, y=w353) -> (x+y=w337:u32)
            n133 = Bundle By Name(cluster=T6 {"ID"=0, "TimeStamp"=0, "TimeFlag"=0, "SendType"=0, "RemoteFlag"=0, "ExternFlag"=0, "DataLen"=0, "Data"=[], "Reserved"=[]} ("Send"), "ID"=w337, "RemoteFlag"=w341, "ExternFlag"=w340, "DataLen"=w345, "Data"=w336) -> (w342:T6)
            n134 = Build Array(w342) -> (w343:T6[])
            n135 = Unbundle By Name(w338) -> ("DevType"=w347:T5, "DevIndex"=w346:u32, "CanIndex"=w344:T4)
            n136 = call "VCI_Transmit.vi"("Buffer"=w343, "CANIndex"=w344, "DevIndex"=w346, "DevType"=w347) -> ()  [unwired: 1 in, 7 out]
          }
          event "电流限制_W": Value Change {
            w374 = u8 0 items=["数据帧", "遥控帧"]
            w375 = u8 0 items=["标准帧", "扩展帧"]
            # "索引地址"
            n137 = event-data() -> ()  [unwired: 2 out]
            n138 = property on="电机ID" class="CmbBox"() -> ("Value"=w366:string)  [unwired: 2 in, 2 out]
            n139 = Multiply ("乘")(x="电流限制", y=i16 8) -> (x*y=w378:i16)
            n140 = Scan From String(format string="%x" ("格式字符串"), input string=w366, default 1=u8 0) -> (output 1=w363:u8)  [unwired: 2 in, 3 out]
            n141 = Absolute Value(x=w378) -> (abs(x)=w380:i16)
            n142 = Add(x=u32 16, y=w363) -> (x+y=w359:u32)
            n143 = Split Number(x=w380) -> (hi(x)=w362:u8, lo(x)=w361:u8)
            n144 = Build Array(u8 87, w362, w361) -> (w358:u8[])
            n145 = Bundle By Name(cluster=T6 {"ID"=0, "TimeStamp"=0, "TimeFlag"=0, "SendType"=0, "RemoteFlag"=0, "ExternFlag"=0, "DataLen"=0, "Data"=[], "Reserved"=[]} ("Send"), "ID"=w359, "RemoteFlag"=w374, "ExternFlag"=w375, "DataLen"=u8 3, "Data"=w358) -> (w373:T6)
            n146 = Build Array(w373) -> (w372:T6[])
            n147 = Unbundle By Name(w360) -> ("DevType"=w369:T5, "DevIndex"=w370:u32, "CanIndex"=w371:T4)
            n148 = call "VCI_Transmit.vi"("Buffer"=w372, "CANIndex"=w371, "DevIndex"=w370, "DevType"=w369) -> ()  [unwired: 1 in, 7 out]
          }
          event "电流限制_R": Value Change {
            w389 = u8 0 items=["数据帧", "遥控帧"]
            w388 = u8 0 items=["标准帧", "扩展帧"]
            # "地址"
            n149 = event-data() -> ()  [unwired: 2 out]
            n150 = property on="电机ID" class="CmbBox"() -> ("Value"=w398:string)  [unwired: 2 in, 2 out]
            n151 = Scan From String(format string="%x" ("格式字符串"), input string=w398, default 1=u8 0) -> (output 1=w401:u8)  [unwired: 2 in, 3 out]
            n152 = call "Demo_MakeData.vi"("DataString"="57 ") -> ("Data"=w384:u8[], "DataLen"=w393:u8)  [unwired: 9 out]
            n153 = Add(x=u32 48, y=w401) -> (x+y=w385:u32)
            n154 = Bundle By Name(cluster=T6 {"ID"=0, "TimeStamp"=0, "TimeFlag"=0, "SendType"=0, "RemoteFlag"=0, "ExternFlag"=0, "DataLen"=0, "Data"=[], "Reserved"=[]} ("Send"), "ID"=w385, "RemoteFlag"=w389, "ExternFlag"=w388, "DataLen"=w393, "Data"=w384) -> (w390:T6)
            n155 = Build Array(w390) -> (w391:T6[])
            n156 = Unbundle By Name(w386) -> ("DevType"=w395:T5, "DevIndex"=w394:u32, "CanIndex"=w392:T4)
            n157 = call "VCI_Transmit.vi"("Buffer"=w391, "CANIndex"=w392, "DevIndex"=w394, "DevType"=w395) -> ()  [unwired: 1 in, 7 out]
          }
          event "监测周期_W": Value Change {
            w420 = u8 0 items=["数据帧", "遥控帧"]
            w421 = u8 0 items=["标准帧", "扩展帧"]
            # "索引地址"
            n158 = event-data() -> ()  [unwired: 2 out]
            n159 = property on="电机ID" class="CmbBox"() -> ("Value"=w412:string)  [unwired: 2 in, 2 out]
            n160 = Scan From String(format string="%x" ("格式字符串"), input string=w412, default 1=u8 0) -> (output 1=w409:u8)  [unwired: 2 in, 3 out]
            n161 = Split Number(x="监测周期") -> (hi(x)=w424:u8, lo(x)=w425:u8)
            n162 = Add(x=u32 16, y=w409) -> (x+y=w407:u32)
            n163 = Build Array(u8 35, w424, w425) -> (w406:u8[])
            n164 = Bundle By Name(cluster=T6 {"ID"=0, "TimeStamp"=0, "TimeFlag"=0, "SendType"=0, "RemoteFlag"=0, "ExternFlag"=0, "DataLen"=0, "Data"=[], "Reserved"=[]} ("Send"), "ID"=w407, "RemoteFlag"=w420, "ExternFlag"=w421, "DataLen"=u8 3, "Data"=w406) -> (w419:T6)
            n165 = Build Array(w419) -> (w418:T6[])
            n166 = Unbundle By Name(w408) -> ("DevType"=w415:T5, "DevIndex"=w416:u32, "CanIndex"=w417:T4)
            n167 = call "VCI_Transmit.vi"("Buffer"=w418, "CANIndex"=w417, "DevIndex"=w416, "DevType"=w415) -> ()  [unwired: 1 in, 7 out]
          }
          event "监测周期_R": Value Change {
            w444 = u8 0 items=["数据帧", "遥控帧"]
            w445 = u8 0 items=["标准帧", "扩展帧"]
            # "地址"
            n168 = event-data() -> ()  [unwired: 2 out]
            n169 = property on="电机ID" class="CmbBox"() -> ("Value"=w435:string)  [unwired: 2 in, 2 out]
            n170 = Scan From String(format string="%x" ("格式字符串"), input string=w435, default 1=u8 0) -> (output 1=w432:u8)  [unwired: 2 in, 3 out]
            n171 = call "Demo_MakeData.vi"("DataString"="23 ") -> ("Data"=w429:u8[], "DataLen"=w440:u8)  [unwired: 9 out]
            n172 = Add(x=u32 48, y=w432) -> (x+y=w430:u32)
            n173 = Bundle By Name(cluster=T6 {"ID"=0, "TimeStamp"=0, "TimeFlag"=0, "SendType"=0, "RemoteFlag"=0, "ExternFlag"=0, "DataLen"=0, "Data"=[], "Reserved"=[]} ("Send"), "ID"=w430, "RemoteFlag"=w444, "ExternFlag"=w445, "DataLen"=w440, "Data"=w429) -> (w443:T6)
            n174 = Build Array(w443) -> (w442:T6[])
            n175 = Unbundle By Name(w431) -> ("DevType"=w438:T5, "DevIndex"=w439:u32, "CanIndex"=w441:T4)
            n176 = call "VCI_Transmit.vi"("Buffer"=w442, "CANIndex"=w441, "DevIndex"=w439, "DevType"=w438) -> ()  [unwired: 1 in, 7 out]
          }
          event "监测_W": Value Change {
            w466 = u8 0 items=["数据帧", "遥控帧"]
            w467 = u8 0 items=["标准帧", "扩展帧"]
            # "地址"
            n177 = event-data() -> ()  [unwired: 2 out]
            n178 = property on="电机ID" class="CmbBox"() -> ("Value"=w455:string)  [unwired: 2 in, 2 out]
            n179 = Scan From String(format string="%x" ("格式字符串"), input string=w455, default 1=u8 0) -> (output 1=w452:u8)  [unwired: 2 in, 3 out]
            n180 = call "Demo_MakeData.vi"("DataString"="监测") -> ("Data"=w450:u8[], "DataLen"=w462:u8)  [unwired: 9 out]
            n181 = Add(x=u32 48, y=w452) -> (x+y=w449:u32)
            n182 = Bundle By Name(cluster=T6 {"ID"=0, "TimeStamp"=0, "TimeFlag"=0, "SendType"=0, "RemoteFlag"=0, "ExternFlag"=0, "DataLen"=0, "Data"=[], "Reserved"=[]} ("Send"), "ID"=w449, "RemoteFlag"=w466, "ExternFlag"=w467, "DataLen"=w462, "Data"=w450) -> (w465:T6)
            n183 = Build Array(w465) -> (w464:T6[])
            n184 = Unbundle By Name(w458) -> ("DevType"=w460:T5, "DevIndex"=w461:u32, "CanIndex"=w463:T4)
            n185 = call "VCI_Transmit.vi"("Buffer"=w464, "CANIndex"=w463, "DevIndex"=w461, "DevType"=w460) -> ()  [unwired: 1 in, 7 out]
          }
          event "看门狗周期_W": Value Change {
            w480 = u8 0 items=["数据帧", "遥控帧"]
            w479 = u8 0 items=["标准帧", "扩展帧"]
            w473 = u32 138
            # "索引地址"
            n186 = event-data() -> ()  [unwired: 2 out]
            n187 = Split Number(x="看门狗周期") -> (hi(x)=w476:u8, lo(x)=w475:u8)
            n188 = Build Array(u8 1, w476, w475) -> (w472:u8[])
            n189 = Bundle By Name(cluster=T6 {"ID"=0, "TimeStamp"=0, "TimeFlag"=0, "SendType"=0, "RemoteFlag"=0, "ExternFlag"=0, "DataLen"=0, "Data"=[], "Reserved"=[]} ("Send"), "ID"=w473, "RemoteFlag"=w480, "ExternFlag"=w479, "DataLen"=u8 3, "Data"=w472) -> (w481:T6)
            n190 = Build Array(w481) -> (w482:T6[])
            n191 = Unbundle By Name(w474) -> ("DevType"=w485:T5, "DevIndex"=w484:u32, "CanIndex"=w483:T4)
            n192 = call "VCI_Transmit.vi"("Buffer"=w482, "CANIndex"=w483, "DevIndex"=w484, "DevType"=w485) -> ()  [unwired: 1 in, 7 out]
          }
          event "看门狗周期_R": Value Change {
            w495 = u8 0 items=["数据帧", "遥控帧"]
            w494 = u8 0 items=["标准帧", "扩展帧"]
            # "地址"
            n193 = event-data() -> ()  [unwired: 2 out]
            n194 = property on="电机ID" class="CmbBox"() -> ("Value"=w504:string)  [unwired: 2 in, 2 out]
            n195 = Scan From String(format string="%x" ("格式字符串"), input string=w504, default 1=u8 0) -> (output 1=w507:u8)  [unwired: 2 in, 3 out]
            n196 = call "Demo_MakeData.vi"("DataString"="01") -> ("Data"=w490:u8[], "DataLen"=w499:u8)  [unwired: 9 out]
            n197 = Add(x=u32 48, y=w507) -> (x+y=w491:u32)
            n198 = Bundle By Name(cluster=T6 {"ID"=0, "TimeStamp"=0, "TimeFlag"=0, "SendType"=0, "RemoteFlag"=0, "ExternFlag"=0, "DataLen"=0, "Data"=[], "Reserved"=[]} ("Send"), "ID"=w491, "RemoteFlag"=w495, "ExternFlag"=w494, "DataLen"=w499, "Data"=w490) -> (w496:T6)
            n199 = Build Array(w496) -> (w497:T6[])
            n200 = Unbundle By Name(w492) -> ("DevType"=w501:T5, "DevIndex"=w500:u32, "CanIndex"=w498:T4)
            n201 = call "VCI_Transmit.vi"("Buffer"=w497, "CANIndex"=w498, "DevIndex"=w500, "DevType"=w501) -> ()  [unwired: 1 in, 7 out]
          }
          event "看门狗_W": Value Change {
            w522 = u8 0 items=["数据帧", "遥控帧"]
            w514 = u32 138
            w523 = u8 0 items=["标准帧", "扩展帧"]
            n202 = event-data() -> ()  [unwired: 2 out]
            n203 = case shown="\"开启\", 默认" "看门狗" {
              tunnel: [w526 w531 w536] -> w511
              frame "开启", Default {
                n204 = Split Number(x=u16 52428) -> (hi(x)=w529:u8, lo(x)=w530:u8)
                n205 = Build Array(u8 2, w529, w530) -> (w526:u8[])
              }
              frame "喂狗" {
                n206 = Split Number(x=u16 43690) -> (hi(x)=w533:u8, lo(x)=w532:u8)
                n207 = Build Array(u8 2, w533, w532) -> (w531:u8[])
              }
              frame "关闭" {
                n208 = Split Number(x=u16 52394) -> (hi(x)=w538:u8, lo(x)=w537:u8)
                n209 = Build Array(u8 2, w538, w537) -> (w536:u8[])
              }
            }
            n210 = Bundle By Name(cluster=T6 {"ID"=0, "TimeStamp"=0, "TimeFlag"=0, "SendType"=0, "RemoteFlag"=0, "ExternFlag"=0, "DataLen"=0, "Data"=[], "Reserved"=[]} ("Send"), "ID"=w514, "RemoteFlag"=w522, "ExternFlag"=w523, "DataLen"=u8 3, "Data"=w511) -> (w521:T6)
            n211 = Build Array(w521) -> (w520:T6[])
            n212 = Unbundle By Name(w515) -> ("DevType"=w517:T5, "DevIndex"=w518:u32, "CanIndex"=w519:T4)
            n213 = call "VCI_Transmit.vi"("Buffer"=w520, "CANIndex"=w519, "DevIndex"=w518, "DevType"=w517) -> ()  [unwired: 1 in, 7 out]
          }
          event "模式_W": Value Change {
            w547 = u8 0 items=["数据帧", "遥控帧"]
            w546 = u8 0 items=["标准帧", "扩展帧"]
            # "地址"
            n214 = event-data() -> ()  [unwired: 2 out]
            n215 = property on="电机ID" class="CmbBox"() -> ("Value"=w556:string)  [unwired: 2 in, 2 out]
            n216 = Concatenate Strings("20 ", "模式") -> (w560:string)
            n217 = Scan From String(format string="%x" ("格式字符串"), input string=w556, default 1=u8 0) -> (output 1=w559:u8)  [unwired: 2 in, 3 out]
            n218 = property on="模式_回" class="CmbBox"("Value"="模式") -> ()  [unwired: 2 in, 2 out]
            n219 = call "Demo_MakeData.vi"("DataString"=w560) -> ("Data"=w543:u8[], "DataLen"=w551:u8)  [unwired: 9 out]
            n220 = Add(x=u32 16, y=w559) -> (x+y=w542:u32)
            n221 = Bundle By Name(cluster=T6 {"ID"=0, "TimeStamp"=0, "TimeFlag"=0, "SendType"=0, "RemoteFlag"=0, "ExternFlag"=0, "DataLen"=0, "Data"=[], "Reserved"=[]} ("Send"), "ID"=w542, "RemoteFlag"=w547, "ExternFlag"=w546, "DataLen"=w551, "Data"=w543) -> (w548:T6)
            n222 = Build Array(w548) -> (w549:T6[])
            n223 = Unbundle By Name(w545) -> ("DevType"=w553:T5, "DevIndex"=w552:u32, "CanIndex"=w550:T4)
            n224 = call "VCI_Transmit.vi"("Buffer"=w549, "CANIndex"=w550, "DevIndex"=w552, "DevType"=w553) -> ()  [unwired: 1 in, 7 out]
          }
          event "模式_R": Value Change {
            w580 = u8 0 items=["数据帧", "遥控帧"]
            w581 = u8 0 items=["标准帧", "扩展帧"]
            # "地址"
            n225 = event-data() -> ()  [unwired: 2 out]
            n226 = property on="电机ID" class="CmbBox"() -> ("Value"=w571:string)  [unwired: 2 in, 2 out]
            n227 = Scan From String(format string="%x" ("格式字符串"), input string=w571, default 1=u8 0) -> (output 1=w568:u8)  [unwired: 2 in, 3 out]
            n228 = call "Demo_MakeData.vi"("DataString"="20 ") -> ("Data"=w565:u8[], "DataLen"=w576:u8)  [unwired: 9 out]
            n229 = Add(x=u32 48, y=w568) -> (x+y=w564:u32)
            n230 = Bundle By Name(cluster=T6 {"ID"=0, "TimeStamp"=0, "TimeFlag"=0, "SendType"=0, "RemoteFlag"=0, "ExternFlag"=0, "DataLen"=0, "Data"=[], "Reserved"=[]} ("Send"), "ID"=w564, "RemoteFlag"=w580, "ExternFlag"=w581, "DataLen"=w576, "Data"=w565) -> (w579:T6)
            n231 = Build Array(w579) -> (w578:T6[])
            n232 = Unbundle By Name(w567) -> ("DevType"=w574:T5, "DevIndex"=w575:u32, "CanIndex"=w577:T4)
            n233 = call "VCI_Transmit.vi"("Buffer"=w578, "CANIndex"=w577, "DevIndex"=w575, "DevType"=w574) -> ()  [unwired: 1 in, 7 out]
          }
          event "设定位置_W": Value Change {
            w597 = u8 0 items=["数据帧", "遥控帧"]
            w596 = u8 0 items=["标准帧", "扩展帧"]
            # "索引地址"
            n234 = event-data() -> ()  [unwired: 2 out]
            n235 = property on="电机ID" class="CmbBox"() -> ("Value"=w605:string)  [unwired: 2 in, 2 out]
            n236 = Multiply ("乘")(x="设定位置", y=u16 256) -> (x*y=w589:i16)
            n237 = Scan From String(format string="%x" ("格式字符串"), input string=w605, default 1=u8 0) -> (output 1=w608:u8)  [unwired: 2 in, 3 out]
            n238 = Split Number(x=w589) -> (hi(x)=w588:u8, lo(x)=w587:u8)
            n239 = Add(x=u32 16, y=w608) -> (x+y=w585:u32)
            n240 = Build Array(u8 64, w588, w587) -> (w586:u8[])
            n241 = Bundle By Name(cluster=T6 {"ID"=0, "TimeStamp"=0, "TimeFlag"=0, "SendType"=0, "RemoteFlag"=0, "ExternFlag"=0, "DataLen"=0, "Data"=[], "Reserved"=[]} ("Send"), "ID"=w585, "RemoteFlag"=w597, "ExternFlag"=w596, "DataLen"=u8 3, "Data"=w586) -> (w598:T6)
            n242 = Build Array(w598) -> (w599:T6[])
            n243 = Unbundle By Name(w595) -> ("DevType"=w602:T5, "DevIndex"=w601:u32, "CanIndex"=w600:T4)
            n244 = call "VCI_Transmit.vi"("Buffer"=w599, "CANIndex"=w600, "DevIndex"=w601, "DevType"=w602) -> ()  [unwired: 1 in, 7 out]
          }
          event "设定速度_W": Value Change {
            w630 = u8 0 items=["数据帧", "遥控帧"]
            w631 = u8 0 items=["标准帧", "扩展帧"]
            # "索引地址"
            n245 = event-data() -> ()  [unwired: 2 out]
            n246 = property on="电机ID" class="CmbBox"() -> ("Value"=w622:string)  [unwired: 2 in, 2 out]
            n247 = Multiply ("乘")(x="设定速度", y=i16 1) -> (x*y=w615:i16)
            n248 = Scan From String(format string="%x" ("格式字符串"), input string=w622, default 1=u8 0) -> (output 1=w619:u8)  [unwired: 2 in, 3 out]
            n249 = Split Number(x=w615) -> (hi(x)=w614:u8, lo(x)=w613:u8)
            n250 = Add(x=u32 16, y=w619) -> (x+y=w611:u32)
            n251 = Build Array(u8 65, w614, w613) -> (w612:u8[])
            n252 = Bundle By Name(cluster=T6 {"ID"=0, "TimeStamp"=0, "TimeFlag"=0, "SendType"=0, "RemoteFlag"=0, "ExternFlag"=0, "DataLen"=0, "Data"=[], "Reserved"=[]} ("Send"), "ID"=w611, "RemoteFlag"=w630, "ExternFlag"=w631, "DataLen"=u8 3, "Data"=w612) -> (w629:T6)
            n253 = Build Array(w629) -> (w628:T6[])
            n254 = Unbundle By Name(w618) -> ("DevType"=w625:T5, "DevIndex"=w626:u32, "CanIndex"=w627:T4)
            n255 = call "VCI_Transmit.vi"("Buffer"=w628, "CANIndex"=w627, "DevIndex"=w626, "DevType"=w625) -> ()  [unwired: 1 in, 7 out]
          }
          event "设定电流_W": Value Change {
            w649 = u8 0 items=["数据帧", "遥控帧"]
            w648 = u8 0 items=["标准帧", "扩展帧"]
            # "索引地址"
            n256 = event-data() -> ()  [unwired: 2 out]
            n257 = property on="电机ID" class="CmbBox"() -> ("Value"=w657:string)  [unwired: 2 in, 2 out]
            n258 = Multiply ("乘")(x="设定电流", y=i16 256) -> (x*y=w641:i16)
            n259 = Scan From String(format string="%x" ("格式字符串"), input string=w657, default 1=u8 0) -> (output 1=w660:u8)  [unwired: 2 in, 3 out]
            n260 = Split Number(x=w641) -> (hi(x)=w640:u8, lo(x)=w639:u8)
            n261 = Add(x=u32 16, y=w660) -> (x+y=w637:u32)
            n262 = Build Array(u8 66, w640, w639) -> (w638:u8[])
            n263 = Bundle By Name(cluster=T6 {"ID"=0, "TimeStamp"=0, "TimeFlag"=0, "SendType"=0, "RemoteFlag"=0, "ExternFlag"=0, "DataLen"=0, "Data"=[], "Reserved"=[]} ("Send"), "ID"=w637, "RemoteFlag"=w649, "ExternFlag"=w648, "DataLen"=u8 3, "Data"=w638) -> (w650:T6)
            n264 = Build Array(w650) -> (w651:T6[])
            n265 = Unbundle By Name(w644) -> ("DevType"=w654:T5, "DevIndex"=w653:u32, "CanIndex"=w652:T4)
            n266 = call "VCI_Transmit.vi"("Buffer"=w651, "CANIndex"=w652, "DevIndex"=w653, "DevType"=w654) -> ()  [unwired: 1 in, 7 out]
          }
          event "电流环KP_W": Value Change {
            w679 = u8 0 items=["数据帧", "遥控帧"]
            w680 = u8 0 items=["标准帧", "扩展帧"]
            # "索引地址"
            n267 = event-data() -> ()  [unwired: 2 out]
            n268 = property on="电机ID" class="CmbBox"() -> ("Value"=w671:string)  [unwired: 2 in, 2 out]
            n269 = Multiply ("乘")(x="电流环KP", y=u16 256) -> (x*y=w684:u16)
            n270 = Scan From String(format string="%x" ("格式字符串"), input string=w671, default 1=u8 0) -> (output 1=w668:u8)  [unwired: 2 in, 3 out]
            n271 = Split Number(x=w684) -> (hi(x)=w685:u8, lo(x)=w686:u8)
            n272 = Add(x=u32 16, y=w668) -> (x+y=w663:u32)
            n273 = Build Array(u8 81, w685, w686) -> (w664:u8[])
            n274 = Bundle By Name(cluster=T6 {"ID"=0, "TimeStamp"=0, "TimeFlag"=0, "SendType"=0, "RemoteFlag"=0, "ExternFlag"=0, "DataLen"=0, "Data"=[], "Reserved"=[]} ("Send"), "ID"=w663, "RemoteFlag"=w679, "ExternFlag"=w680, "DataLen"=u8 3, "Data"=w664) -> (w678:T6)
            n275 = Build Array(w678) -> (w677:T6[])
            n276 = Unbundle By Name(w667) -> ("DevType"=w674:T5, "DevIndex"=w675:u32, "CanIndex"=w676:T4)
            n277 = call "VCI_Transmit.vi"("Buffer"=w677, "CANIndex"=w676, "DevIndex"=w675, "DevType"=w674) -> ()  [unwired: 1 in, 7 out]
          }
          event "电流环KI_W": Value Change {
            w701 = u8 0 items=["数据帧", "遥控帧"]
            w700 = u8 0 items=["标准帧", "扩展帧"]
            # "索引地址"
            n278 = event-data() -> ()  [unwired: 2 out]
            n279 = property on="电机ID" class="CmbBox"() -> ("Value"=w709:string)  [unwired: 2 in, 2 out]
            n280 = Multiply ("乘")(x="电流环KI", y=u16 256) -> (x*y=w696:u16)
            n281 = Scan From String(format string="%x" ("格式字符串"), input string=w709, default 1=u8 0) -> (output 1=w712:u8)  [unwired: 2 in, 3 out]
            n282 = Split Number(x=w696) -> (hi(x)=w695:u8, lo(x)=w694:u8)
            n283 = Add(x=u32 16, y=w712) -> (x+y=w689:u32)
            n284 = Build Array(u8 82, w695, w694) -> (w690:u8[])
            n285 = Bundle By Name(cluster=T6 {"ID"=0, "TimeStamp"=0, "TimeFlag"=0, "SendType"=0, "RemoteFlag"=0, "ExternFlag"=0, "DataLen"=0, "Data"=[], "Reserved"=[]} ("Send"), "ID"=w689, "RemoteFlag"=w701, "ExternFlag"=w700, "DataLen"=u8 3, "Data"=w690) -> (w702:T6)
            n286 = Build Array(w702) -> (w703:T6[])
            n287 = Unbundle By Name(w693) -> ("DevType"=w706:T5, "DevIndex"=w705:u32, "CanIndex"=w704:T4)
            n288 = call "VCI_Transmit.vi"("Buffer"=w703, "CANIndex"=w704, "DevIndex"=w705, "DevType"=w706) -> ()  [unwired: 1 in, 7 out]
          }
          event "速度环KP_W": Value Change {
            w727 = u8 0 items=["数据帧", "遥控帧"]
            w726 = u8 0 items=["标准帧", "扩展帧"]
            # "索引地址"
            n289 = event-data() -> ()  [unwired: 2 out]
            n290 = property on="电机ID" class="CmbBox"() -> ("Value"=w735:string)  [unwired: 2 in, 2 out]
            n291 = Multiply ("乘")(x="速度环KP", y=u16 256) -> (x*y=w722:u16)
            n292 = Scan From String(format string="%x" ("格式字符串"), input string=w735, default 1=u8 0) -> (output 1=w738:u8)  [unwired: 2 in, 3 out]
            n293 = Split Number(x=w722) -> (hi(x)=w721:u8, lo(x)=w720:u8)
            n294 = Add(x=u32 16, y=w738) -> (x+y=w715:u32)
            n295 = Build Array(u8 83, w721, w720) -> (w716:u8[])
            n296 = Bundle By Name(cluster=T6 {"ID"=0, "TimeStamp"=0, "TimeFlag"=0, "SendType"=0, "RemoteFlag"=0, "ExternFlag"=0, "DataLen"=0, "Data"=[], "Reserved"=[]} ("Send"), "ID"=w715, "RemoteFlag"=w727, "ExternFlag"=w726, "DataLen"=u8 3, "Data"=w716) -> (w728:T6)
            n297 = Build Array(w728) -> (w729:T6[])
            n298 = Unbundle By Name(w719) -> ("DevType"=w732:T5, "DevIndex"=w731:u32, "CanIndex"=w730:T4)
            n299 = call "VCI_Transmit.vi"("Buffer"=w729, "CANIndex"=w730, "DevIndex"=w731, "DevType"=w732) -> ()  [unwired: 1 in, 7 out]
          }
          event "速度环KI_W": Value Change {
            w757 = u8 0 items=["数据帧", "遥控帧"]
            w758 = u8 0 items=["标准帧", "扩展帧"]
            # "索引地址"
            n300 = event-data() -> ()  [unwired: 2 out]
            n301 = property on="电机ID" class="CmbBox"() -> ("Value"=w749:string)  [unwired: 2 in, 2 out]
            n302 = Multiply ("乘")(x="速度环KI", y=u16 256) -> (x*y=w762:u16)
            n303 = Scan From String(format string="%x" ("格式字符串"), input string=w749, default 1=u8 0) -> (output 1=w746:u8)  [unwired: 2 in, 3 out]
            n304 = Split Number(x=w762) -> (hi(x)=w763:u8, lo(x)=w764:u8)
            n305 = Add(x=u32 16, y=w746) -> (x+y=w741:u32)
            n306 = Build Array(u8 84, w763, w764) -> (w742:u8[])
            n307 = Bundle By Name(cluster=T6 {"ID"=0, "TimeStamp"=0, "TimeFlag"=0, "SendType"=0, "RemoteFlag"=0, "ExternFlag"=0, "DataLen"=0, "Data"=[], "Reserved"=[]} ("Send"), "ID"=w741, "RemoteFlag"=w757, "ExternFlag"=w758, "DataLen"=u8 3, "Data"=w742) -> (w756:T6)
            n308 = Build Array(w756) -> (w755:T6[])
            n309 = Unbundle By Name(w745) -> ("DevType"=w752:T5, "DevIndex"=w753:u32, "CanIndex"=w754:T4)
            n310 = call "VCI_Transmit.vi"("Buffer"=w755, "CANIndex"=w754, "DevIndex"=w753, "DevType"=w752) -> ()  [unwired: 1 in, 7 out]
          }
          event "加速度_W": Value Change {
            w779 = u8 0 items=["数据帧", "遥控帧"]
            w778 = u8 0 items=["标准帧", "扩展帧"]
            # "索引地址"
            n311 = event-data() -> ()  [unwired: 2 out]
            n312 = property on="电机ID" class="CmbBox"() -> ("Value"=w787:string)  [unwired: 2 in, 2 out]
            n313 = Multiply ("乘")(x="加速度", y=u16 8) -> (x*y=w774:u16)
            n314 = Scan From String(format string="%x" ("格式字符串"), input string=w787, default 1=u8 0) -> (output 1=w790:u8)  [unwired: 2 in, 3 out]
            n315 = Split Number(x=w774) -> (hi(x)=w773:u8, lo(x)=w772:u8)
            n316 = Add(x=u32 16, y=w790) -> (x+y=w767:u32)
            n317 = Build Array(u8 85, w773, w772) -> (w768:u8[])
            n318 = Bundle By Name(cluster=T6 {"ID"=0, "TimeStamp"=0, "TimeFlag"=0, "SendType"=0, "RemoteFlag"=0, "ExternFlag"=0, "DataLen"=0, "Data"=[], "Reserved"=[]} ("Send"), "ID"=w767, "RemoteFlag"=w779, "ExternFlag"=w778, "DataLen"=u8 3, "Data"=w768) -> (w780:T6)
            n319 = Build Array(w780) -> (w781:T6[])
            n320 = Unbundle By Name(w771) -> ("DevType"=w784:T5, "DevIndex"=w783:u32, "CanIndex"=w782:T4)
            n321 = call "VCI_Transmit.vi"("Buffer"=w781, "CANIndex"=w782, "DevIndex"=w783, "DevType"=w784) -> ()  [unwired: 1 in, 7 out]
          }
          event "减速度_W": Value Change {
            w809 = u8 0 items=["数据帧", "遥控帧"]
            w810 = u8 0 items=["标准帧", "扩展帧"]
            # "索引地址"
            n322 = event-data() -> ()  [unwired: 2 out]
            n323 = property on="电机ID" class="CmbBox"() -> ("Value"=w801:string)  [unwired: 2 in, 2 out]
            n324 = Multiply ("乘")(x="减速度", y=u16 8) -> (x*y=w814:u16)
            n325 = Scan From String(format string="%x" ("格式字符串"), input string=w801, default 1=u8 0) -> (output 1=w798:u8)  [unwired: 2 in, 3 out]
            n326 = Split Number(x=w814) -> (hi(x)=w815:u8, lo(x)=w816:u8)
            n327 = Add(x=u32 16, y=w798) -> (x+y=w794:u32)
            n328 = Build Array(u8 86, w815, w816) -> (w795:u8[])
            n329 = Bundle By Name(cluster=T6 {"ID"=0, "TimeStamp"=0, "TimeFlag"=0, "SendType"=0, "RemoteFlag"=0, "ExternFlag"=0, "DataLen"=0, "Data"=[], "Reserved"=[]} ("Send"), "ID"=w794, "RemoteFlag"=w809, "ExternFlag"=w810, "DataLen"=u8 3, "Data"=w795) -> (w808:T6)
            n330 = Build Array(w808) -> (w807:T6[])
            n331 = Unbundle By Name(w797) -> ("DevType"=w804:T5, "DevIndex"=w805:u32, "CanIndex"=w806:T4)
            n332 = call "VCI_Transmit.vi"("Buffer"=w807, "CANIndex"=w806, "DevIndex"=w805, "DevType"=w804) -> ()  [unwired: 1 in, 7 out]
          }
          event "AI_K0_W": Value Change {
            w829 = u8 0 items=["数据帧", "遥控帧"]
            w828 = u8 0 items=["标准帧", "扩展帧"]
            # "索引地址"
            n333 = event-data() -> ()  [unwired: 2 out]
            n334 = property on="电机ID" class="CmbBox"() -> ("Value"=w837:string)  [unwired: 2 in, 2 out]
            n335 = Scan From String(format string="%x" ("格式字符串"), input string=w837, default 1=u8 0) -> (output 1=w840:u8)  [unwired: 2 in, 3 out]
            n336 = Split Number(x="A电流零偏") -> (hi(x)=w825:u8, lo(x)=w824:u8)
            n337 = Add(x=u32 16, y=w840) -> (x+y=w819:u32)
            n338 = Build Array(u8 90, w825, w824) -> (w820:u8[])
            n339 = Bundle By Name(cluster=T6 {"ID"=0, "TimeStamp"=0, "TimeFlag"=0, "SendType"=0, "RemoteFlag"=0, "ExternFlag"=0, "DataLen"=0, "Data"=[], "Reserved"=[]} ("Send"), "ID"=w819, "RemoteFlag"=w829, "ExternFlag"=w828, "DataLen"=u8 3, "Data"=w820) -> (w830:T6)
            n340 = Build Array(w830) -> (w831:T6[])
            n341 = Unbundle By Name(w823) -> ("DevType"=w834:T5, "DevIndex"=w833:u32, "CanIndex"=w832:T4)
            n342 = call "VCI_Transmit.vi"("Buffer"=w831, "CANIndex"=w832, "DevIndex"=w833, "DevType"=w834) -> ()  [unwired: 1 in, 7 out]
          }
          event "BI_K0_W": Value Change {
            w853 = u8 0 items=["数据帧", "遥控帧"]
            w852 = u8 0 items=["标准帧", "扩展帧"]
            # "索引地址"
            n343 = event-data() -> ()  [unwired: 2 out]
            n344 = property on="电机ID" class="CmbBox"() -> ("Value"=w861:string)  [unwired: 2 in, 2 out]
            n345 = Scan From String(format string="%x" ("格式字符串"), input string=w861, default 1=u8 0) -> (output 1=w864:u8)  [unwired: 2 in, 3 out]
            n346 = Split Number(x="B电流零偏") -> (hi(x)=w849:u8, lo(x)=w848:u8)
            n347 = Add(x=u32 16, y=w864) -> (x+y=w843:u32)
            n348 = Build Array(u8 91, w849, w848) -> (w844:u8[])
            n349 = Bundle By Name(cluster=T6 {"ID"=0, "TimeStamp"=0, "TimeFlag"=0, "SendType"=0, "RemoteFlag"=0, "ExternFlag"=0, "DataLen"=0, "Data"=[], "Reserved"=[]} ("Send"), "ID"=w843, "RemoteFlag"=w853, "ExternFlag"=w852, "DataLen"=u8 3, "Data"=w844) -> (w854:T6)
            n350 = Build Array(w854) -> (w855:T6[])
            n351 = Unbundle By Name(w847) -> ("DevType"=w858:T5, "DevIndex"=w857:u32, "CanIndex"=w856:T4)
            n352 = call "VCI_Transmit.vi"("Buffer"=w855, "CANIndex"=w856, "DevIndex"=w857, "DevType"=w858) -> ()  [unwired: 1 in, 7 out]
          }
          event "CI_K0_W": Value Change {
            w877 = u8 0 items=["数据帧", "遥控帧"]
            w876 = u8 0 items=["标准帧", "扩展帧"]
            # "索引地址"
            n353 = event-data() -> ()  [unwired: 2 out]
            n354 = property on="电机ID" class="CmbBox"() -> ("Value"=w885:string)  [unwired: 2 in, 2 out]
            n355 = Scan From String(format string="%x" ("格式字符串"), input string=w885, default 1=u8 0) -> (output 1=w888:u8)  [unwired: 2 in, 3 out]
            n356 = Split Number(x="C电流零偏") -> (hi(x)=w873:u8, lo(x)=w872:u8)
            n357 = Add(x=u32 16, y=w888) -> (x+y=w867:u32)
            n358 = Build Array(u8 92, w873, w872) -> (w868:u8[])
            n359 = Bundle By Name(cluster=T6 {"ID"=0, "TimeStamp"=0, "TimeFlag"=0, "SendType"=0, "RemoteFlag"=0, "ExternFlag"=0, "DataLen"=0, "Data"=[], "Reserved"=[]} ("Send"), "ID"=w867, "RemoteFlag"=w877, "ExternFlag"=w876, "DataLen"=u8 3, "Data"=w868) -> (w878:T6)
            n360 = Build Array(w878) -> (w879:T6[])
            n361 = Unbundle By Name(w871) -> ("DevType"=w882:T5, "DevIndex"=w881:u32, "CanIndex"=w880:T4)
            n362 = call "VCI_Transmit.vi"("Buffer"=w879, "CANIndex"=w880, "DevIndex"=w881, "DevType"=w882) -> ()  [unwired: 1 in, 7 out]
          }
          event "对准角_W": Value Change {
            w910 = u8 0 items=["数据帧", "遥控帧"]
            w911 = u8 0 items=["标准帧", "扩展帧"]
            # "索引地址"
            n363 = event-data() -> ()  [unwired: 2 out]
            n364 = property on="电机ID" class="CmbBox"() -> ("Value"=w902:string)  [unwired: 2 in, 2 out]
            n365 = Multiply(x="对准角", y=u16 8) -> (x*y=w893:dbl)
            n366 = Scan From String(format string="%x" ("格式字符串"), input string=w902, default 1=u8 0) -> (output 1=w899:u8)  [unwired: 2 in, 3 out]
            n367 = To Unsigned Word Integer(number=w893) -> (unsigned 16bit integer=w892:u16)
            n368 = Add(x=u32 16, y=w899) -> (x+y=w897:u32)
            n369 = Split Number(x=w892) -> (hi(x)=w914:u8, lo(x)=w915:u8)
            n370 = Build Array(u8 93, w914, w915) -> (w896:u8[])
            n371 = Bundle By Name(cluster=T6 {"ID"=0, "TimeStamp"=0, "TimeFlag"=0, "SendType"=0, "RemoteFlag"=0, "ExternFlag"=0, "DataLen"=0, "Data"=[], "Reserved"=[]} ("Send"), "ID"=w897, "RemoteFlag"=w910, "ExternFlag"=w911, "DataLen"=u8 3, "Data"=w896) -> (w909:T6)
            n372 = Build Array(w909) -> (w908:T6[])
            n373 = Unbundle By Name(w898) -> ("DevType"=w905:T5, "DevIndex"=w906:u32, "CanIndex"=w907:T4)
            n374 = call "VCI_Transmit.vi"("Buffer"=w908, "CANIndex"=w907, "DevIndex"=w906, "DevType"=w905) -> ()  [unwired: 1 in, 7 out]
          }
          event "DATA_SAVE_W": Value Change {
            w934 = u8 0 items=["数据帧", "遥控帧"]
            w935 = u8 0 items=["标准帧", "扩展帧"]
            # "地址"
            n375 = event-data() -> ()  [unwired: 2 out]
            n376 = property on="电机ID" class="CmbBox"() -> ("Value"=w925:string)  [unwired: 2 in, 2 out]
            n377 = Scan From String(format string="%x" ("格式字符串"), input string=w925, default 1=u8 0) -> (output 1=w922:u8)  [unwired: 2 in, 3 out]
            n378 = call "Demo_MakeData.vi"("DataString"="50") -> ("Data"=w919:u8[], "DataLen"=w930:u8)  [unwired: 9 out]
            n379 = Add(x=u32 16, y=w922) -> (x+y=w918:u32)
            n380 = Bundle By Name(cluster=T6 {"ID"=0, "TimeStamp"=0, "TimeFlag"=0, "SendType"=0, "RemoteFlag"=0, "ExternFlag"=0, "DataLen"=0, "Data"=[], "Reserved"=[]} ("Send"), "ID"=w918, "RemoteFlag"=w934, "ExternFlag"=w935, "DataLen"=w930, "Data"=w919) -> (w933:T6)
            n381 = Build Array(w933) -> (w932:T6[])
            n382 = Unbundle By Name(w921) -> ("DevType"=w928:T5, "DevIndex"=w929:u32, "CanIndex"=w931:T4)
            n383 = call "VCI_Transmit.vi"("Buffer"=w932, "CANIndex"=w931, "DevIndex"=w929, "DevType"=w928) -> ()  [unwired: 1 in, 7 out]
          }
          event "设定位置_R": Value Change {
            w945 = u8 0 items=["数据帧", "遥控帧"]
            w944 = u8 0 items=["标准帧", "扩展帧"]
            # "地址"
            n384 = event-data() -> ()  [unwired: 2 out]
            n385 = property on="电机ID" class="CmbBox"() -> ("Value"=w954:string)  [unwired: 2 in, 2 out]
            n386 = Scan From String(format string="%x" ("格式字符串"), input string=w954, default 1=u8 0) -> (output 1=w957:u8)  [unwired: 2 in, 3 out]
            n387 = call "Demo_MakeData.vi"("DataString"="40 ") -> ("Data"=w940:u8[], "DataLen"=w949:u8)  [unwired: 9 out]
            n388 = Add(x=u32 48, y=w957) -> (x+y=w939:u32)
            n389 = Bundle By Name(cluster=T6 {"ID"=0, "TimeStamp"=0, "TimeFlag"=0, "SendType"=0, "RemoteFlag"=0, "ExternFlag"=0, "DataLen"=0, "Data"=[], "Reserved"=[]} ("Send"), "ID"=w939, "RemoteFlag"=w945, "ExternFlag"=w944, "DataLen"=w949, "Data"=w940) -> (w946:T6)
            n390 = Build Array(w946) -> (w947:T6[])
            n391 = Unbundle By Name(w942) -> ("DevType"=w951:T5, "DevIndex"=w950:u32, "CanIndex"=w948:T4)
            n392 = call "VCI_Transmit.vi"("Buffer"=w947, "CANIndex"=w948, "DevIndex"=w950, "DevType"=w951) -> ()  [unwired: 1 in, 7 out]
          }
          event "设定速度_R": Value Change {
            w976 = u8 0 items=["数据帧", "遥控帧"]
            w977 = u8 0 items=["标准帧", "扩展帧"]
            # "地址"
            n393 = event-data() -> ()  [unwired: 2 out]
            n394 = property on="电机ID" class="CmbBox"() -> ("Value"=w967:string)  [unwired: 2 in, 2 out]
            n395 = Scan From String(format string="%x" ("格式字符串"), input string=w967, default 1=u8 0) -> (output 1=w964:u8)  [unwired: 2 in, 3 out]
            n396 = call "Demo_MakeData.vi"("DataString"="41 ") -> ("Data"=w961:u8[], "DataLen"=w972:u8)  [unwired: 9 out]
            n397 = Add(x=u32 48, y=w964) -> (x+y=w960:u32)
            n398 = Bundle By Name(cluster=T6 {"ID"=0, "TimeStamp"=0, "TimeFlag"=0, "SendType"=0, "RemoteFlag"=0, "ExternFlag"=0, "DataLen"=0, "Data"=[], "Reserved"=[]} ("Send"), "ID"=w960, "RemoteFlag"=w976, "ExternFlag"=w977, "DataLen"=w972, "Data"=w961) -> (w975:T6)
            n399 = Build Array(w975) -> (w974:T6[])
            n400 = Unbundle By Name(w963) -> ("DevType"=w970:T5, "DevIndex"=w971:u32, "CanIndex"=w973:T4)
            n401 = call "VCI_Transmit.vi"("Buffer"=w974, "CANIndex"=w973, "DevIndex"=w971, "DevType"=w970) -> ()  [unwired: 1 in, 7 out]
          }
          event "设定电流_R": Value Change {
            w997 = u8 0 items=["数据帧", "遥控帧"]
            w998 = u8 0 items=["标准帧", "扩展帧"]
            # "地址"
            n402 = event-data() -> ()  [unwired: 2 out]
            n403 = property on="电机ID" class="CmbBox"() -> ("Value"=w988:string)  [unwired: 2 in, 2 out]
            n404 = Scan From String(format string="%x" ("格式字符串"), input string=w988, default 1=u8 0) -> (output 1=w985:u8)  [unwired: 2 in, 3 out]
            n405 = call "Demo_MakeData.vi"("DataString"="42 ") -> ("Data"=w982:u8[], "DataLen"=w993:u8)  [unwired: 9 out]
            n406 = Add(x=u32 48, y=w985) -> (x+y=w981:u32)
            n407 = Bundle By Name(cluster=T6 {"ID"=0, "TimeStamp"=0, "TimeFlag"=0, "SendType"=0, "RemoteFlag"=0, "ExternFlag"=0, "DataLen"=0, "Data"=[], "Reserved"=[]} ("Send"), "ID"=w981, "RemoteFlag"=w997, "ExternFlag"=w998, "DataLen"=w993, "Data"=w982) -> (w996:T6)
            n408 = Build Array(w996) -> (w995:T6[])
            n409 = Unbundle By Name(w984) -> ("DevType"=w991:T5, "DevIndex"=w992:u32, "CanIndex"=w994:T4)
            n410 = call "VCI_Transmit.vi"("Buffer"=w995, "CANIndex"=w994, "DevIndex"=w992, "DevType"=w991) -> ()  [unwired: 1 in, 7 out]
          }
          event "电流环KP_R": Value Change {
            w1018 = u8 0 items=["数据帧", "遥控帧"]
            w1019 = u8 0 items=["标准帧", "扩展帧"]
            # "地址"
            n411 = event-data() -> ()  [unwired: 2 out]
            n412 = property on="电机ID" class="CmbBox"() -> ("Value"=w1009:string)  [unwired: 2 in, 2 out]
            n413 = Scan From String(format string="%x" ("格式字符串"), input string=w1009, default 1=u8 0) -> (output 1=w1006:u8)  [unwired: 2 in, 3 out]
            n414 = call "Demo_MakeData.vi"("DataString"="51 ") -> ("Data"=w1003:u8[], "DataLen"=w1014:u8)  [unwired: 9 out]
            n415 = Add(x=u32 48, y=w1006) -> (x+y=w1002:u32)
            n416 = Bundle By Name(cluster=T6 {"ID"=0, "TimeStamp"=0, "TimeFlag"=0, "SendType"=0, "RemoteFlag"=0, "ExternFlag"=0, "DataLen"=0, "Data"=[], "Reserved"=[]} ("Send"), "ID"=w1002, "RemoteFlag"=w1018, "ExternFlag"=w1019, "DataLen"=w1014, "Data"=w1003) -> (w1017:T6)
            n417 = Build Array(w1017) -> (w1016:T6[])
            n418 = Unbundle By Name(w1005) -> ("DevType"=w1012:T5, "DevIndex"=w1013:u32, "CanIndex"=w1015:T4)
            n419 = call "VCI_Transmit.vi"("Buffer"=w1016, "CANIndex"=w1015, "DevIndex"=w1013, "DevType"=w1012) -> ()  [unwired: 1 in, 7 out]
          }
          event "电流环KI_R": Value Change {
            w1039 = u8 0 items=["数据帧", "遥控帧"]
            w1040 = u8 0 items=["标准帧", "扩展帧"]
            # "地址"
            n420 = event-data() -> ()  [unwired: 2 out]
            n421 = property on="电机ID" class="CmbBox"() -> ("Value"=w1030:string)  [unwired: 2 in, 2 out]
            n422 = Scan From String(format string="%x" ("格式字符串"), input string=w1030, default 1=u8 0) -> (output 1=w1027:u8)  [unwired: 2 in, 3 out]
            n423 = call "Demo_MakeData.vi"("DataString"="52 ") -> ("Data"=w1024:u8[], "DataLen"=w1035:u8)  [unwired: 9 out]
            n424 = Add(x=u32 48, y=w1027) -> (x+y=w1023:u32)
            n425 = Bundle By Name(cluster=T6 {"ID"=0, "TimeStamp"=0, "TimeFlag"=0, "SendType"=0, "RemoteFlag"=0, "ExternFlag"=0, "DataLen"=0, "Data"=[], "Reserved"=[]} ("Send"), "ID"=w1023, "RemoteFlag"=w1039, "ExternFlag"=w1040, "DataLen"=w1035, "Data"=w1024) -> (w1038:T6)
            n426 = Build Array(w1038) -> (w1037:T6[])
            n427 = Unbundle By Name(w1026) -> ("DevType"=w1033:T5, "DevIndex"=w1034:u32, "CanIndex"=w1036:T4)
            n428 = call "VCI_Transmit.vi"("Buffer"=w1037, "CANIndex"=w1036, "DevIndex"=w1034, "DevType"=w1033) -> ()  [unwired: 1 in, 7 out]
          }
          event "速度环KP_R": Value Change {
            w1050 = u8 0 items=["数据帧", "遥控帧"]
            w1049 = u8 0 items=["标准帧", "扩展帧"]
            # "地址"
            n429 = event-data() -> ()  [unwired: 2 out]
            n430 = property on="电机ID" class="CmbBox"() -> ("Value"=w1059:string)  [unwired: 2 in, 2 out]
            n431 = Scan From String(format string="%x" ("格式字符串"), input string=w1059, default 1=u8 0) -> (output 1=w1062:u8)  [unwired: 2 in, 3 out]
            n432 = call "Demo_MakeData.vi"("DataString"="53 ") -> ("Data"=w1045:u8[], "DataLen"=w1054:u8)  [unwired: 9 out]
            n433 = Add(x=u32 48, y=w1062) -> (x+y=w1044:u32)
            n434 = Bundle By Name(cluster=T6 {"ID"=0, "TimeStamp"=0, "TimeFlag"=0, "SendType"=0, "RemoteFlag"=0, "ExternFlag"=0, "DataLen"=0, "Data"=[], "Reserved"=[]} ("Send"), "ID"=w1044, "RemoteFlag"=w1050, "ExternFlag"=w1049, "DataLen"=w1054, "Data"=w1045) -> (w1051:T6)
            n435 = Build Array(w1051) -> (w1052:T6[])
            n436 = Unbundle By Name(w1047) -> ("DevType"=w1056:T5, "DevIndex"=w1055:u32, "CanIndex"=w1053:T4)
            n437 = call "VCI_Transmit.vi"("Buffer"=w1052, "CANIndex"=w1053, "DevIndex"=w1055, "DevType"=w1056) -> ()  [unwired: 1 in, 7 out]
          }
          event "速度环KI_R": Value Change {
            w1071 = u8 0 items=["数据帧", "遥控帧"]
            w1070 = u8 0 items=["标准帧", "扩展帧"]
            # "地址"
            n438 = event-data() -> ()  [unwired: 2 out]
            n439 = property on="电机ID" class="CmbBox"() -> ("Value"=w1080:string)  [unwired: 2 in, 2 out]
            n440 = Scan From String(format string="%x" ("格式字符串"), input string=w1080, default 1=u8 0) -> (output 1=w1083:u8)  [unwired: 2 in, 3 out]
            n441 = call "Demo_MakeData.vi"("DataString"="54 ") -> ("Data"=w1066:u8[], "DataLen"=w1075:u8)  [unwired: 9 out]
            n442 = Add(x=u32 48, y=w1083) -> (x+y=w1065:u32)
            n443 = Bundle By Name(cluster=T6 {"ID"=0, "TimeStamp"=0, "TimeFlag"=0, "SendType"=0, "RemoteFlag"=0, "ExternFlag"=0, "DataLen"=0, "Data"=[], "Reserved"=[]} ("Send"), "ID"=w1065, "RemoteFlag"=w1071, "ExternFlag"=w1070, "DataLen"=w1075, "Data"=w1066) -> (w1072:T6)
            n444 = Build Array(w1072) -> (w1073:T6[])
            n445 = Unbundle By Name(w1068) -> ("DevType"=w1077:T5, "DevIndex"=w1076:u32, "CanIndex"=w1074:T4)
            n446 = call "VCI_Transmit.vi"("Buffer"=w1073, "CANIndex"=w1074, "DevIndex"=w1076, "DevType"=w1077) -> ()  [unwired: 1 in, 7 out]
          }
          event "加速度_R": Value Change {
            w1102 = u8 0 items=["数据帧", "遥控帧"]
            w1103 = u8 0 items=["标准帧", "扩展帧"]
            # "地址"
            n447 = event-data() -> ()  [unwired: 2 out]
            n448 = property on="电机ID" class="CmbBox"() -> ("Value"=w1093:string)  [unwired: 2 in, 2 out]
            n449 = Scan From String(format string="%x" ("格式字符串"), input string=w1093, default 1=u8 0) -> (output 1=w1090:u8)  [unwired: 2 in, 3 out]
            n450 = call "Demo_MakeData.vi"("DataString"="55") -> ("Data"=w1087:u8[], "DataLen"=w1098:u8)  [unwired: 9 out]
            n451 = Add(x=u32 48, y=w1090) -> (x+y=w1086:u32)
            n452 = Bundle By Name(cluster=T6 {"ID"=0, "TimeStamp"=0, "TimeFlag"=0, "SendType"=0, "RemoteFlag"=0, "ExternFlag"=0, "DataLen"=0, "Data"=[], "Reserved"=[]} ("Send"), "ID"=w1086, "RemoteFlag"=w1102, "ExternFlag"=w1103, "DataLen"=w1098, "Data"=w1087) -> (w1101:T6)
            n453 = Build Array(w1101) -> (w1100:T6[])
            n454 = Unbundle By Name(w1089) -> ("DevType"=w1096:T5, "DevIndex"=w1097:u32, "CanIndex"=w1099:T4)
            n455 = call "VCI_Transmit.vi"("Buffer"=w1100, "CANIndex"=w1099, "DevIndex"=w1097, "DevType"=w1096) -> ()  [unwired: 1 in, 7 out]
          }
          event "减速度_R": Value Change {
            w1113 = u8 0 items=["数据帧", "遥控帧"]
            w1112 = u8 0 items=["标准帧", "扩展帧"]
            # "地址"
            n456 = event-data() -> ()  [unwired: 2 out]
            n457 = property on="电机ID" class="CmbBox"() -> ("Value"=w1122:string)  [unwired: 2 in, 2 out]
            n458 = Scan From String(format string="%x" ("格式字符串"), input string=w1122, default 1=u8 0) -> (output 1=w1125:u8)  [unwired: 2 in, 3 out]
            n459 = call "Demo_MakeData.vi"("DataString"="56") -> ("Data"=w1108:u8[], "DataLen"=w1117:u8)  [unwired: 9 out]
            n460 = Add(x=u32 48, y=w1125) -> (x+y=w1109:u32)
            n461 = Bundle By Name(cluster=T6 {"ID"=0, "TimeStamp"=0, "TimeFlag"=0, "SendType"=0, "RemoteFlag"=0, "ExternFlag"=0, "DataLen"=0, "Data"=[], "Reserved"=[]} ("Send"), "ID"=w1109, "RemoteFlag"=w1113, "ExternFlag"=w1112, "DataLen"=w1117, "Data"=w1108) -> (w1114:T6)
            n462 = Build Array(w1114) -> (w1115:T6[])
            n463 = Unbundle By Name(w1110) -> ("DevType"=w1119:T5, "DevIndex"=w1118:u32, "CanIndex"=w1116:T4)
            n464 = call "VCI_Transmit.vi"("Buffer"=w1115, "CANIndex"=w1116, "DevIndex"=w1118, "DevType"=w1119) -> ()  [unwired: 1 in, 7 out]
          }
          event "AI_K0_R": Value Change {
            w1134 = u8 0 items=["数据帧", "遥控帧"]
            w1133 = u8 0 items=["标准帧", "扩展帧"]
            # "地址"
            n465 = event-data() -> ()  [unwired: 2 out]
            n466 = property on="电机ID" class="CmbBox"() -> ("Value"=w1143:string)  [unwired: 2 in, 2 out]
            n467 = Scan From String(format string="%x" ("格式字符串"), input string=w1143, default 1=u8 0) -> (output 1=w1146:u8)  [unwired: 2 in, 3 out]
            n468 = call "Demo_MakeData.vi"("DataString"="5A") -> ("Data"=w1129:u8[], "DataLen"=w1138:u8)  [unwired: 9 out]
            n469 = Add(x=u32 48, y=w1146) -> (x+y=w1128:u32)
            n470 = Bundle By Name(cluster=T6 {"ID"=0, "TimeStamp"=0, "TimeFlag"=0, "SendType"=0, "RemoteFlag"=0, "ExternFlag"=0, "DataLen"=0, "Data"=[], "Reserved"=[]} ("Send"), "ID"=w1128, "RemoteFlag"=w1134, "ExternFlag"=w1133, "DataLen"=w1138, "Data"=w1129) -> (w1135:T6)
            n471 = Build Array(w1135) -> (w1136:T6[])
            n472 = Unbundle By Name(w1131) -> ("DevType"=w1140:T5, "DevIndex"=w1139:u32, "CanIndex"=w1137:T4)
            n473 = call "VCI_Transmit.vi"("Buffer"=w1136, "CANIndex"=w1137, "DevIndex"=w1139, "DevType"=w1140) -> ()  [unwired: 1 in, 7 out]
          }
          event "BI_K0_R": Value Change {
            w1155 = u8 0 items=["数据帧", "遥控帧"]
            w1154 = u8 0 items=["标准帧", "扩展帧"]
            # "地址"
            n474 = event-data() -> ()  [unwired: 2 out]
            n475 = property on="电机ID" class="CmbBox"() -> ("Value"=w1164:string)  [unwired: 2 in, 2 out]
            n476 = Scan From String(format string="%x" ("格式字符串"), input string=w1164, default 1=u8 0) -> (output 1=w1167:u8)  [unwired: 2 in, 3 out]
            n477 = call "Demo_MakeData.vi"("DataString"="5B") -> ("Data"=w1150:u8[], "DataLen"=w1159:u8)  [unwired: 9 out]
            n478 = Add(x=u32 48, y=w1167) -> (x+y=w1149:u32)
            n479 = Bundle By Name(cluster=T6 {"ID"=0, "TimeStamp"=0, "TimeFlag"=0, "SendType"=0, "RemoteFlag"=0, "ExternFlag"=0, "DataLen"=0, "Data"=[], "Reserved"=[]} ("Send"), "ID"=w1149, "RemoteFlag"=w1155, "ExternFlag"=w1154, "DataLen"=w1159, "Data"=w1150) -> (w1156:T6)
            n480 = Build Array(w1156) -> (w1157:T6[])
            n481 = Unbundle By Name(w1152) -> ("DevType"=w1161:T5, "DevIndex"=w1160:u32, "CanIndex"=w1158:T4)
            n482 = call "VCI_Transmit.vi"("Buffer"=w1157, "CANIndex"=w1158, "DevIndex"=w1160, "DevType"=w1161) -> ()  [unwired: 1 in, 7 out]
          }
          event "CI_K0_R": Value Change {
            w1176 = u8 0 items=["数据帧", "遥控帧"]
            w1175 = u8 0 items=["标准帧", "扩展帧"]
            # "地址"
            n483 = event-data() -> ()  [unwired: 2 out]
            n484 = property on="电机ID" class="CmbBox"() -> ("Value"=w1185:string)  [unwired: 2 in, 2 out]
            n485 = Scan From String(format string="%x" ("格式字符串"), input string=w1185, default 1=u8 0) -> (output 1=w1188:u8)  [unwired: 2 in, 3 out]
            n486 = call "Demo_MakeData.vi"("DataString"="5C") -> ("Data"=w1171:u8[], "DataLen"=w1180:u8)  [unwired: 9 out]
            n487 = Add(x=u32 48, y=w1188) -> (x+y=w1170:u32)
            n488 = Bundle By Name(cluster=T6 {"ID"=0, "TimeStamp"=0, "TimeFlag"=0, "SendType"=0, "RemoteFlag"=0, "ExternFlag"=0, "DataLen"=0, "Data"=[], "Reserved"=[]} ("Send"), "ID"=w1170, "RemoteFlag"=w1176, "ExternFlag"=w1175, "DataLen"=w1180, "Data"=w1171) -> (w1177:T6)
            n489 = Build Array(w1177) -> (w1178:T6[])
            n490 = Unbundle By Name(w1173) -> ("DevType"=w1182:T5, "DevIndex"=w1181:u32, "CanIndex"=w1179:T4)
            n491 = call "VCI_Transmit.vi"("Buffer"=w1178, "CANIndex"=w1179, "DevIndex"=w1181, "DevType"=w1182) -> ()  [unwired: 1 in, 7 out]
          }
          event "对准角_R": Value Change {
            w1207 = u8 0 items=["数据帧", "遥控帧"]
            w1208 = u8 0 items=["标准帧", "扩展帧"]
            # "地址"
            n492 = event-data() -> ()  [unwired: 2 out]
            n493 = property on="电机ID" class="CmbBox"() -> ("Value"=w1198:string)  [unwired: 2 in, 2 out]
            n494 = Scan From String(format string="%x" ("格式字符串"), input string=w1198, default 1=u8 0) -> (output 1=w1195:u8)  [unwired: 2 in, 3 out]
            n495 = call "Demo_MakeData.vi"("DataString"="5D") -> ("Data"=w1192:u8[], "DataLen"=w1203:u8)  [unwired: 9 out]
            n496 = Add(x=u32 48, y=w1195) -> (x+y=w1193:u32)
            n497 = Bundle By Name(cluster=T6 {"ID"=0, "TimeStamp"=0, "TimeFlag"=0, "SendType"=0, "RemoteFlag"=0, "ExternFlag"=0, "DataLen"=0, "Data"=[], "Reserved"=[]} ("Send"), "ID"=w1193, "RemoteFlag"=w1207, "ExternFlag"=w1208, "DataLen"=w1203, "Data"=w1192) -> (w1206:T6)
            n498 = Build Array(w1206) -> (w1205:T6[])
            n499 = Unbundle By Name(w1194) -> ("DevType"=w1201:T5, "DevIndex"=w1202:u32, "CanIndex"=w1204:T4)
            n500 = call "VCI_Transmit.vi"("Buffer"=w1205, "CANIndex"=w1204, "DevIndex"=w1202, "DevType"=w1201) -> ()  [unwired: 1 in, 7 out]
          }
          event "保存": Value Change {
            w1235 = "-"
            n501 = event-data() -> ()  [unwired: 2 out]
            n502 = Get Date/Time String(want seconds? (F)=TRUE) -> (date string=w1215:string, time string=w1236:string)  [unwired: 2 in]
            n503 = Search and Replace String(input string=w1215, search string="/", replace string="-") -> (result string=w1221:string)  [unwired: 5 in, 3 out]
            n504 = Search and Replace String(input string=w1236, search string=":", replace string="-") -> (result string=w1233:string)  [unwired: 5 in, 3 out]
            n505 = property on="保存_S" class="Bool (严格)"() -> ("Value"=w1227:bool)  [unwired: 2 in, 2 out]
            n506 = Search and Replace String(input string=w1221, search string="/", replace string="-") -> (result string=w1216:string)  [unwired: 5 in, 3 out]
            n507 = Search and Replace String(input string=w1233, search string=":", replace string="-") -> (result string=w1234:string)  [unwired: 5 in, 3 out]
            n508 = Not(x=w1227) -> (.not. x?=w1223:bool)
            n509 = property on="保存_S" class="Bool (严格)"("Value"=w1223) -> ()  [unwired: 2 in, 2 out]
            n510 = Concatenate Strings("D:\\PMSM\\", w1216, w1235, w1234, w1235, "电机数据存储", ".txt") -> (w1213:string)
            n511 = Select(t=w1213, s=w1223, f="") -> (s? t:f=w1228:string)
            n512 = String To Path(string=w1228) -> (path=w1214:path)
            n513 = local write "存储路径"(w1214) -> ()
          }
          event "Close": Value Change {
            w1248 = T10 1 items=["OK"=1, "ERROR1"=0, "ERROR2"=-1] ("y")
            n514 = event-data() -> ()  [unwired: 2 out]
            n515 = Unbundle By Name(w1252) -> ("DevType"=w1251:T5, "DevIndex"=w1250:u32)
            n516 = call "VCI_CloseDevice.vi"("DevIndex"=w1250, "DevType"=w1251) -> ("Return Val"=w1249:T10)  [unwired: 1 in, 8 out]
            n517 = Equal?(x=w1249, y=w1248) -> (x = y?=w1246:bool)
            n518 = Not(x=w1246) -> (.not. x?=w1242:bool)
            n519 = Bundle By Name(cluster=cluster{"CANOpen":bool} {"CANOpen"=FALSE} ("事件数据"), "CANOpen"=w1242) -> (w1241:cluster{"CANOpen":bool})
            n520 = Bundle By Name(cluster=w1247, "Open"=w1242) -> (w1245:cluster{"Open":bool, "SendCnt":u32})
            n521 = local write "Open"(w1242) -> ()
            n522 = Generate User Event(user event=w1244, event data cluster=w1241) -> ()  [unwired: 1 in, 2 out]
          }
          event User Event {
            w1263 = u8 0
            w1262 = u8 2
            n523 = event-data() -> ("CANOpen"=w1256:bool)  [unwired: 1 out]
            "Open" <- w1256
            n524 = Not(x=w1256) -> (.not. x?=w1257:bool)
            n525 = Select(t=w1262, s=w1256, f=w1263) -> (s? t:f=w1255:u8)
            n526 = Select(t=w1263, s=w1256, f=w1262) -> (s? t:f=w1254:u8)
            n527 = property class="VI"("Front Panel.Closeable"=w1257) -> ()  [unwired: 2 in, 2 out]
            n528 = property on="Close" class="Bool"("DisabledEnum"=w1254) -> ()  [unwired: 2 in, 2 out]
            n529 = property on="ID" class="DigNum (严格)"("DisabledEnum"=w1254) -> ()  [unwired: 2 in, 2 out]
            n530 = property on="Data" class="Str"("DisabledEnum"=w1254) -> ()  [unwired: 2 in, 2 out]
            n531 = property on="Format" class="Ring (严格)"("DisabledEnum"=w1254) -> ()  [unwired: 2 in, 2 out]
            n532 = property on="Type" class="Ring (严格)"("DisabledEnum"=w1254) -> ()  [unwired: 2 in, 2 out]
            n533 = property on="Send" class="Bool"("DisabledEnum"=w1254) -> ()  [unwired: 2 in, 2 out]
            n534 = Select(t=enum16{"Init", "Wait", "Run", "Exit"}."Run", s=w1256, f=enum16{"Init", "Wait", "Run", "Exit"}."Wait") -> (s? t:f=w1259:enum16{"Init", "Wait", "Run", "Exit"})
            n535 = property on="Fliter" class="Ring (严格)"("DisabledEnum"=w1255) -> ()  [unwired: 2 in, 2 out]
            n536 = property on="DevType" class="Ring (严格)"("DisabledEnum"=w1255) -> ()  [unwired: 2 in, 2 out]
            n537 = property on="Channel" class="Ring (严格)"("DisabledEnum"=w1255) -> ()  [unwired: 2 in, 2 out]
            n538 = property on="AccCode" class="DigNum (严格)"("DisabledEnum"=w1255) -> ()  [unwired: 2 in, 2 out]
            n539 = property on="AccMask" class="DigNum (严格)"("DisabledEnum"=w1255) -> ()  [unwired: 2 in, 2 out]
            n540 = property on="InitFlag" class="Ring (严格)"("DisabledEnum"=w1255) -> ()  [unwired: 2 in, 2 out]
            n541 = property on="Mode" class="Ring (严格)"("DisabledEnum"=w1255) -> ()  [unwired: 2 in, 2 out]
            n542 = property on="kBaudRate" class="Ring (严格)"("DisabledEnum"=w1255) -> ()  [unwired: 2 in, 2 out]
            n543 = property on="电机ID_W" class="Bool"("DisabledEnum"=w1254) -> ()  [unwired: 2 in, 2 out]
            n544 = property on="监测_W" class="Bool"("DisabledEnum"=w1254) -> ()  [unwired: 2 in, 2 out]
            n545 = property on="模式_W" class="Bool"("DisabledEnum"=w1254) -> ()  [unwired: 2 in, 2 out]
            n546 = property on="模式_R" class="Bool"("DisabledEnum"=w1254) -> ()  [unwired: 2 in, 2 out]
            n547 = property on="设定位置_W" class="Bool"("DisabledEnum"=w1254) -> ()  [unwired: 2 in, 2 out]
            n548 = property on="设定位置_R" class="Bool"("DisabledEnum"=w1254) -> ()  [unwired: 2 in, 2 out]
            n549 = property on="设定速度_W" class="Bool"("DisabledEnum"=w1254) -> ()  [unwired: 2 in, 2 out]
            n550 = property on="设定速度_R" class="Bool"("DisabledEnum"=w1254) -> ()  [unwired: 2 in, 2 out]
            n551 = property on="设定电流_W" class="Bool"("DisabledEnum"=w1254) -> ()  [unwired: 2 in, 2 out]
            n552 = property on="设定电流_R" class="Bool"("DisabledEnum"=w1254) -> ()  [unwired: 2 in, 2 out]
            n553 = property on="保存" class="Bool"("DisabledEnum"=w1254) -> ()  [unwired: 2 in, 2 out]
            n554 = property on="电流环KP_W" class="Bool"("DisabledEnum"=w1254) -> ()  [unwired: 2 in, 2 out]
            n555 = property on="电流环KI_W" class="Bool"("DisabledEnum"=w1254) -> ()  [unwired: 2 in, 2 out]
            n556 = property on="速度环KP_W" class="Bool"("DisabledEnum"=w1254) -> ()  [unwired: 2 in, 2 out]
            n557 = property on="速度环KI_W" class="Bool"("DisabledEnum"=w1254) -> ()  [unwired: 2 in, 2 out]
            n558 = property on="加速度_W" class="Bool"("DisabledEnum"=w1254) -> ()  [unwired: 2 in, 2 out]
            n559 = property on="AI_K0_W" class="Bool"("DisabledEnum"=w1254) -> ()  [unwired: 2 in, 2 out]
            n560 = property on="BI_K0_W" class="Bool"("DisabledEnum"=w1254) -> ()  [unwired: 2 in, 2 out]
            n561 = property on="CI_K0_W" class="Bool"("DisabledEnum"=w1254) -> ()  [unwired: 2 in, 2 out]
            n562 = property on="DATA_SAVE_W" class="Bool"("DisabledEnum"=w1254) -> ()  [unwired: 2 in, 2 out]
            n563 = property on="监测周期_W" class="Bool"("DisabledEnum"=w1254) -> ()  [unwired: 2 in, 2 out]
            n564 = property on="看门狗_W" class="Bool"("DisabledEnum"=w1254) -> ()  [unwired: 2 in, 2 out]
            n565 = property on="电流环KP_R" class="Bool"("DisabledEnum"=w1254) -> ()  [unwired: 2 in, 2 out]
            n566 = property on="电流环KI_R" class="Bool"("DisabledEnum"=w1254) -> ()  [unwired: 2 in, 2 out]
            n567 = property on="速度环KP_R" class="Bool"("DisabledEnum"=w1254) -> ()  [unwired: 2 in, 2 out]
            n568 = property on="速度环KI_R" class="Bool"("DisabledEnum"=w1254) -> ()  [unwired: 2 in, 2 out]
            n569 = property on="加速度_R" class="Bool"("DisabledEnum"=w1254) -> ()  [unwired: 2 in, 2 out]
            n570 = property on="AI_K0_R" class="Bool"("DisabledEnum"=w1254) -> ()  [unwired: 2 in, 2 out]
            n571 = property on="BI_K0_R" class="Bool"("DisabledEnum"=w1254) -> ()  [unwired: 2 in, 2 out]
            n572 = property on="CI_K0_R" class="Bool"("DisabledEnum"=w1254) -> ()  [unwired: 2 in, 2 out]
            n573 = property on="监测周期_R" class="Bool"("DisabledEnum"=w1254) -> ()  [unwired: 2 in, 2 out]
            n574 = property on="看门狗周期_W" class="Bool"("DisabledEnum"=w1254) -> ()  [unwired: 2 in, 2 out]
            n575 = property on="看门狗周期_R" class="Bool"("DisabledEnum"=w1254) -> ()  [unwired: 2 in, 2 out]
            n576 = property on="减速度_R" class="Bool"("DisabledEnum"=w1254) -> ()  [unwired: 2 in, 2 out]
            n577 = property on="减速度_W" class="Bool"("DisabledEnum"=w1254) -> ()  [unwired: 2 in, 2 out]
            n578 = property on="对准角_W" class="Bool"("DisabledEnum"=w1254) -> ()  [unwired: 2 in, 2 out]
            n579 = property on="对准角_R" class="Bool"("DisabledEnum"=w1254) -> ()  [unwired: 2 in, 2 out]
            n580 = property on="电机校准_W" class="Bool"("DisabledEnum"=w1254) -> ()  [unwired: 2 in, 2 out]
            n581 = property on="极对数_W" class="Bool"("DisabledEnum"=w1254) -> ()  [unwired: 2 in, 2 out]
            n582 = property on="极对数_R" class="Bool"("DisabledEnum"=w1254) -> ()  [unwired: 2 in, 2 out]
            n583 = property on="编码器线数_W" class="Bool"("DisabledEnum"=w1254) -> ()  [unwired: 2 in, 2 out]
            n584 = property on="编码器线数_R" class="Bool"("DisabledEnum"=w1254) -> ()  [unwired: 2 in, 2 out]
            n585 = property on="速度限制_W" class="Bool"("DisabledEnum"=w1254) -> ()  [unwired: 2 in, 2 out]
            n586 = property on="速度限制_R" class="Bool"("DisabledEnum"=w1254) -> ()  [unwired: 2 in, 2 out]
            n587 = property on="电流限制_W" class="Bool"("DisabledEnum"=w1254) -> ()  [unwired: 2 in, 2 out]
            n588 = property on="电流限制_R" class="Bool"("DisabledEnum"=w1254) -> ()  [unwired: 2 in, 2 out]
          }
        }
        "数组" <- w150
        "CAN ID" <- w149
      }
      frame "Exit" {
        n589 = Release Queue(queue=w1274) -> ()  [unwired: 1 in, 4 out]
        n590 = Unregister For Events(event registration refnum=w1273) -> (error out=w1272:errorcluster)  [unwired: 1 in]
        n591 = Destroy User Event(user event=w1271, error in=w1272) -> ()  [unwired: 1 out]
        n592 = Unbundle By Name(w1270) -> ("Open"=w1269:bool)
        n593 = case shown="真" w1269 {
          tunnel: w1268 -> [_ w1278]
          frame False {
          }
          frame True {
            n594 = Unbundle By Name(w1278) -> ("DevType"=w1277:T5, "DevIndex"=w1276:u32)
            n595 = call "VCI_CloseDevice.vi"("DevIndex"=w1276, "DevType"=w1277) -> ()  [unwired: 1 in, 9 out]
          }
        }
        n596 = local write "RcvEnable"(FALSE ("RcvEnable")) -> ()
      }
    }
  }
  n597 = while "数据更新线程" {
    tunnel: w9 -> [w1284]
    shift-right: [w1279] -> _
    shift-left: u32 0 ("RecvCnt") -> [w1280]
    stop <- w1283 stop-if-true
    n598 = Dequeue Element(queue=w1284) -> (element=w1282:T7, timed out?=w1281:bool, error out=w1283:errorcluster)  [unwired: 2 in, 1 out]
    n599 = case shown="假" w1281 {
      tunnel: w1282 -> [w1294 _]
      tunnel: w1280 -> [w1288 w1709]
      tunnel: [w1287 w1709] -> w1279
      frame False {
        n600 = Array To Cluster(array=w1294) -> (cluster=w1296:T12)
        n601 = Unbundle By Name(w1296) -> ("[0]"=w1295:T13)
        n602 = Increment(x=w1288) -> (x+1=w1287:u32)
        "sCnt" <- w1287
        n603 = Unbundle By Name(w1295) -> ("VCI_CAN_OBJ"=w1293:T6)  [unwired: 3 out]
        n604 = Unbundle By Name(w1293) -> ("ID"=w1291:u32, "Data"=w1292:u8[])  [unwired: 7 out]
        "CAN STD_ID" <- w1291
        n605 = And(x=w1291, y=u32 15) -> (x .and. y?=→"电机ID_R":u32)
        n606 = And(x=w1291, y=u32 240) -> (x .and. y?=w1286:u32)
        n607 = case shown="40" w1286 {
          tunnel: w1292 -> [_ w1302]
          frame 0, Default {
          }
          frame 64 {
            n608 = local read "存储路径"() -> (w1298:path)
            n609 = local read "保存_S"() -> (w1299:bool)
            n610 = Index Array(array=w1302, index=0) -> (element=w1301:u8)
            n611 = case shown="58" w1301 {
              tunnel: w1302 -> [_ w1327 w1336 w1349 w1360 w1367 w1385 w1405 w1429 w1446 w1466 w1479 w1504 w1523 w1540 w1544 w1551 w1559 w1569 w1575 w1588 w1591 w1601 w1611 w1621 w1631 w1641 w1651 w1661 w1669 w1678 w1681 w1687 w1695 w1701 w1704]
              tunnel: [_ _ _ _ _ _ w1373 w1395 w1418 w1444 w1461 w1478 w1493 w1517 _ _ _ _ _ _ _ _ _ _ _ _ _ _ _ _ _ _ _ _ _ _] -> w1297
              frame 0, Default {
              }
              frame 1 {
                n612 = Array To Cluster(array=w1327) -> (cluster=w1328:T14)
                n613 = Unbundle By Name(w1328) -> ("Data[1]"=w1330:u8, "Data[2]"=w1331:u8)  [unwired: 1 out]
                n614 = Join Numbers(hi=w1330, lo=w1331) -> ((hi.lo)=w1329:u16)
                n615 = To Unsigned Word Integer(number=w1329) -> (unsigned 16bit integer=→"看门狗周期_回":u16)
              }
              frame 32 {
                n616 = Array To Cluster(array=w1336) -> (cluster=w1337:T14)
                n617 = Unbundle By Name(w1337) -> ("Data[1]"=w1335:u8)  [unwired: 1 out]
                n618 = To Unsigned Byte Integer(number=w1335) -> (unsigned 8bit integer=w1332:u8)
                n619 = Number To Hexadecimal String(1:2, 2:w1332) -> (0:w1333:string)
                n620 = property on="模式_回" class="CmbBox"("Value"=w1333) -> ()  [unwired: 2 in, 2 out]
              }
              frame 33 {
                n621 = Array To Cluster(array=w1349) -> (cluster=w1351:T14)
                n622 = Unbundle By Name(w1351) -> ("Data[1]"=w1350:u8)  [unwired: 1 out]
                n623 = To Unsigned Byte Integer(number=w1350) -> (unsigned 8bit integer=w1348:u8)
                n624 = Number To Boolean Array(number=w1348) -> (Boolean array=w1347:bool[])
                n625 = Array To Cluster(array=w1347) -> (cluster=w1346:T15)
                n626 = Unbundle(w1346) -> ("Boolean array[0]"=→"warn0":bool, "Boolean array[1]"=→"warn1":bool, "Boolean array[2]"=→"高温":bool, "Boolean array[3]"=→"warn3":bool, "Boolean array[4]"=→"warn4":bool, "Boolean array[5]"=→"warn5":bool, "Boolean array[6]"=→"warn6":bool, "Boolean array[7]"=→"warn7":bool)
              }
              frame 34 {
                n627 = Array To Cluster(array=w1360) -> (cluster=w1365:T14)
                n628 = Unbundle By Name(w1365) -> ("Data[1]"=w1364:u8)  [unwired: 1 out]
                n629 = To Unsigned Byte Integer(number=w1364) -> (unsigned 8bit integer=w1363:u8)
                n630 = Number To Boolean Array(number=w1363) -> (Boolean array=w1362:bool[])
                n631 = Array To Cluster(array=w1362) -> (cluster=w1361:T15)
                n632 = Unbundle(w1361) -> ("Boolean array[0]"=→"低压":bool, "Boolean array[1]"=→"高压":bool, "Boolean array[2]"=→"高温":bool, "Boolean array[3]"=→"ERRO3":bool, "Boolean array[4]"=→"ERRO4":bool, "Boolean array[5]"=→"ERRO5":bool, "Boolean array[6]"=→"ERRO6":bool, "Boolean array[7]"=→"ERRO7":bool)
              }
              frame 35 {
                n633 = Array To Cluster(array=w1367) -> (cluster=w1368:T14)
                n634 = Unbundle By Name(w1368) -> ("Data[1]"=w1370:u8, "Data[2]"=w1371:u8)  [unwired: 1 out]
                n635 = Join Numbers(hi=w1370, lo=w1371) -> ((hi.lo)=w1369:u16)
                n636 = To Unsigned Word Integer(number=w1369) -> (unsigned 16bit integer=→"监测周期_回":u16)
              }
              frame 49 {
                w1374 = 0.0054931640625
                w1387 = 8
                n637 = Array To Cluster(array=w1385) -> (cluster=w1391:T14)
                n638 = Unbundle By Name(w1391) -> ("Data[1]"=w1379:u8, "Data[2]"=w1380:u8, "Data[3]"=w1381:u8, "Data[4]"=w1382:u8, "Data[5]"=w1378:u8, "Data[6]"=w1377:u8)  [unwired: 1 out]
                n639 = Join Numbers(hi=w1378, lo=w1377) -> ((hi.lo)=w1376:u16)
                n640 = To Unsigned Word Integer(number=w1379) -> (unsigned 16bit integer=w1394:u16)
                n641 = To Unsigned Word Integer(number=w1381) -> (unsigned 16bit integer=w1390:u16)
                n642 = To Word Integer(number=w1376) -> (16bit integer=w1375:i16)
                n643 = Rotate(1:w1394, 2:w1387) -> (0:w1393:u16)
                n644 = Rotate(1:w1390, 2:w1387) -> (0:w1389:u16)
                n645 = Add(x=w1393, y=w1380) -> (x+y=w1392:u16)
                n646 = Add(x=w1389, y=w1382) -> (x+y=w1388:u16)
                n647 = Multiply(x=w1392, y=w1374) -> (x*y=w1384:dbl)
                "机械角度" <- w1384
                n648 = Multiply(x=w1388, y=w1374) -> (x*y=w1383:dbl)
                "电气角度" <- w1383
                n649 = Divide(x=w1375, y=1.0) -> (x/y=w1372:dbl)
                "转速" <- w1372
                "转速" <- w1372
                n650 = Build Array(w1384, w1383, w1372) -> (w1373:dbl[])
              }
              frame 50 {
                w1406 = i16 1024
                w1407 = 8
                n651 = Array To Cluster(array=w1405) -> (cluster=w1414:T14)
                n652 = Unbundle By Name(w1414) -> ("Data[1]"=w1404:u8, "Data[2]"=w1403:u8, "Data[3]"=w1402:u8, "Data[4]"=w1401:u8, "Data[5]"=w1400:u8, "Data[6]"=w1399:u8)  [unwired: 1 out]
                n653 = To Word Integer(number=w1404) -> (16bit integer=w1417:i16)
                n654 = To Word Integer(number=w1400) -> (16bit integer=w1410:i16)
                n655 = To Word Integer(number=w1402) -> (16bit integer=w1413:i16)
                n656 = Rotate(1:w1417, 2:w1407) -> (0:w1416:i16)
                n657 = Rotate(1:w1410, 2:w1407) -> (0:w1409:i16)
                n658 = Rotate(1:w1413, 2:w1407) -> (0:w1412:i16)
                n659 = Add(x=w1416, y=w1403) -> (x+y=w1415:i16)
                n660 = Add(x=w1409, y=w1399) -> (x+y=w1408:i16)
                n661 = Add(x=w1412, y=w1401) -> (x+y=w1411:i16)
                n662 = Divide(x=w1415, y=w1406) -> (x/y=w1398:dbl)
                "A电流" <- w1398
                "波形图表1" <- w1398
                n663 = Divide(x=w1408, y=w1406) -> (x/y=w1396:dbl)
                "C电流" <- w1396
                "波形图表3" <- w1396
                n664 = Divide(x=w1411, y=w1406) -> (x/y=w1397:dbl)
                "B电流" <- w1397
                "波形图表2" <- w1397
                n665 = Build Array(w1398, w1397, w1396) -> (w1395:dbl[])
              }
              frame 51 {
                w1431 = i16 256
                w1430 = 8
                n666 = Array To Cluster(array=w1429) -> (cluster=w1438:T14)
                n667 = Unbundle By Name(w1438) -> ("Data[1]"=w1428:u8, "Data[2]"=w1427:u8, "Data[3]"=w1426:u8, "Data[4]"=w1425:u8, "Data[5]"=w1424:u8, "Data[6]"=w1423:u8)  [unwired: 1 out]
                n668 = To Unsigned Word Integer(number=w1428) -> (unsigned 16bit integer=w1441:u16)
                n669 = To Word Integer(number=w1426) -> (16bit integer=w1437:i16)
                n670 = To Word Integer(number=w1424) -> (16bit integer=w1434:i16)
                n671 = Rotate(1:w1441, 2:w1430) -> (0:w1440:u16)
                n672 = Rotate(1:w1437, 2:w1430) -> (0:w1436:i16)
                n673 = Rotate(1:w1434, 2:w1430) -> (0:w1433:i16)
                n674 = Add(x=w1440, y=w1427) -> (x+y=w1439:u16)
                n675 = Add(x=w1436, y=w1425) -> (x+y=w1435:i16)
                n676 = Add(x=w1433, y=w1423) -> (x+y=w1432:i16)
                n677 = Divide(x=w1439, y=i16 1024) -> (x/y=w1421:dbl)
                "供电电压" <- w1421
                n678 = Divide(x=w1435, y=w1431) -> (x/y=w1420:dbl)
                "Ialfa" <- w1420
                n679 = Divide(x=w1432, y=w1431) -> (x/y=w1419:dbl)
                "Ibeta" <- w1419
                n680 = Build Array(w1421, w1420, w1419) -> (w1418:dbl[])
              }
              frame 52 {
                w1445 = i16 256
                w1451 = 8
                n681 = Array To Cluster(array=w1446) -> (cluster=w1455:T14)
                n682 = Unbundle By Name(w1455) -> ("Data[1]"=w1450:u8, "Data[2]"=w1449:u8, "Data[3]"=w1448:u8, "Data[4]"=w1447:u8)  [unwired: 1 out]
                n683 = To Word Integer(number=w1450) -> (16bit integer=w1458:i16)
                n684 = To Word Integer(number=w1448) -> (16bit integer=w1454:i16)
                n685 = Rotate(1:w1458, 2:w1451) -> (0:w1457:i16)
                n686 = Rotate(1:w1454, 2:w1451) -> (0:w1453:i16)
                n687 = Add(x=w1457, y=w1449) -> (x+y=w1456:i16)
                n688 = Add(x=w1453, y=w1447) -> (x+y=w1452:i16)
                n689 = Divide(x=w1456, y=w1445) -> (x/y=w1443:dbl)
                "Iqnow" <- w1443
                n690 = Divide(x=w1452, y=w1445) -> (x/y=w1442:dbl)
                "Idnow" <- w1442
                n691 = Build Array(w1443, w1442) -> (w1444:dbl[])
              }
              frame 53 {
                w1468 = i16 1024
                w1467 = 8
                n692 = Array To Cluster(array=w1466) -> (cluster=w1472:T14)
                n693 = Unbundle By Name(w1472) -> ("Data[1]"=w1465:u8, "Data[2]"=w1464:u8, "Data[3]"=w1463:u8, "Data[4]"=w1462:u8)  [unwired: 1 out]
                n694 = To Word Integer(number=w1465) -> (16bit integer=w1475:i16)
                n695 = To Word Integer(number=w1463) -> (16bit integer=w1471:i16)
                n696 = Rotate(1:w1475, 2:w1467) -> (0:w1474:i16)
                n697 = Rotate(1:w1471, 2:w1467) -> (0:w1470:i16)
                n698 = Add(x=w1474, y=w1464) -> (x+y=w1473:i16)
                n699 = Add(x=w1470, y=w1462) -> (x+y=w1469:i16)
                n700 = Divide(x=w1473, y=w1468) -> (x/y=w1460:dbl)
                "Uq" <- w1460
                n701 = Divide(x=w1469, y=w1468) -> (x/y=w1459:dbl)
                "Ud" <- w1459
                n702 = Build Array(w1460, w1459) -> (w1461:dbl[])
              }
              frame 54 {
                w1485 = i16 1024
                w1484 = 8
                n703 = Array To Cluster(array=w1479) -> (cluster=w1489:T14)
                n704 = Unbundle By Name(w1489) -> ("Data[1]"=w1483:u8, "Data[2]"=w1482:u8, "Data[3]"=w1481:u8, "Data[4]"=w1480:u8)  [unwired: 1 out]
                n705 = To Word Integer(number=w1483) -> (16bit integer=w1492:i16)
                n706 = To Word Integer(number=w1481) -> (16bit integer=w1488:i16)
                n707 = Rotate(1:w1492, 2:w1484) -> (0:w1491:i16)
                n708 = Rotate(1:w1488, 2:w1484) -> (0:w1487:i16)
                n709 = Add(x=w1491, y=w1482) -> (x+y=w1490:i16)
                n710 = Add(x=w1487, y=w1480) -> (x+y=w1486:i16)
                n711 = Divide(x=w1490, y=w1485) -> (x/y=w1477:dbl)
                "Ualfa" <- w1477
                n712 = Divide(x=w1486, y=w1485) -> (x/y=w1476:dbl)
                "Ubate" <- w1476
                n713 = Build Array(w1477, w1476) -> (w1478:dbl[])
              }
              frame 55 {
                w1506 = u16 0
                w1505 = 8
                n714 = Array To Cluster(array=w1504) -> (cluster=w1513:T14)
                n715 = Unbundle By Name(w1513) -> ("Data[1]"=w1498:u8, "Data[2]"=w1499:u8, "Data[3]"=w1500:u8, "Data[4]"=w1501:u8, "Data[5]"=w1502:u8, "Data[6]"=w1503:u8, "Data[7]"=w1494:u8)  [unwired: 1 out]
                "sector" <- w1494
                n716 = To Word Integer(number=w1498) -> (16bit integer=w1516:i16)
                n717 = To Word Integer(number=w1500) -> (16bit integer=w1512:i16)
                n718 = To Word Integer(number=w1502) -> (16bit integer=w1509:i16)
                n719 = Rotate(1:w1516, 2:w1505) -> (0:w1515:i16)
                n720 = Rotate(1:w1512, 2:w1505) -> (0:w1511:i16)
                n721 = Rotate(1:w1509, 2:w1505) -> (0:w1508:i16)
                n722 = Add(x=w1515, y=w1499) -> (x+y=w1514:i16)
                n723 = Add(x=w1511, y=w1501) -> (x+y=w1510:i16)
                n724 = Add(x=w1508, y=w1503) -> (x+y=w1507:i16)
                n725 = Subtract ("减")(x=w1514, y=w1506) -> (x-y=w1497:u16)
                "PWM1" <- w1497
                n726 = Subtract ("减")(x=w1510, y=w1506) -> (x-y=w1496:u16)
                "PWM2" <- w1496
                n727 = Subtract ("减")(x=w1507, y=w1506) -> (x-y=w1495:u16)
                "PWM3" <- w1495
                n728 = Build Array(w1497, w1496, w1495, w1494) -> (w1493:u16[])
              }
              frame 56 {
                n729 = Array Subset(array=w1523, index=1, length=4) -> (w1520:u8[])
                n730 = Type Cast(type=2097152, x=w1520) -> (*(type *) &x=w1518:i32)
                "Sin" <- w1518
                "Cosin" <- w1518
                n731 = Build Array(w1518, w1518) -> (w1517:i32[])
              }
              frame 57 {
                n732 = Array To Cluster(array=w1540) -> (cluster=w1541:cluster{"Data[0]":u8, "Data[1]":u8})
                n733 = Unbundle By Name(w1541) -> ("Data[1]"=w1532:u8)  [unwired: 1 out]
                n734 = And(x=w1532, y=u8 56) -> (x .and. y?=w1535:u8)
                n735 = And(x=w1532, y=u8 192) -> (x .and. y?=w1538:u8)
                n736 = And(x=w1532, y=u8 7) -> (x .and. y?=w1529:u8)
                n737 = Logical Shift(y=i16 -3, x=w1535) -> (x << y=w1531:u8)
                n738 = Logical Shift(y=i16 -6, x=w1538) -> (x << y=w1527:u8)
                n739 = Divide(x=w1531, y=u8 10) -> (x/y=w1526:dbl)
                n740 = Divide(x=w1529, y=u8 100) -> (x/y=w1525:dbl)
                n741 = Compound Arithmetic op=ADD(w1527, w1526, w1525) -> (→"版本号":dbl)
              }
              frame 58 {
                n742 = Array To Cluster(array=w1544) -> (cluster=w1549:T14)
                n743 = Unbundle By Name(w1549) -> ("Data[1]"=w1547:u8, "Data[2]"=w1546:u8)  [unwired: 1 out]
                n744 = Join Numbers(hi=w1547, lo=w1546) -> ((hi.lo)=w1548:u16)
                n745 = To Unsigned Word Integer(number=w1548) -> (unsigned 16bit integer=w1545:u16)
                n746 = Multiply(x=w1545, y=0.0054931640625) -> (x*y=w1543:dbl)
                n747 = property on="机械角度" class="DigNum (严格)"("Value"=w1543) -> ()  [unwired: 2 in, 2 out]
              }
              frame 59 {
                n748 = Array To Cluster(array=w1551) -> (cluster=w1557:T14)
                n749 = Unbundle By Name(w1557) -> ("Data[1]"=w1555:u8, "Data[2]"=w1554:u8)  [unwired: 1 out]
                n750 = Join Numbers(hi=w1555, lo=w1554) -> ((hi.lo)=w1556:u16)
                n751 = To Word Integer(number=w1556) -> (16bit integer=w1553:i16)
                n752 = Divide(x=w1553, y=i16 1) -> (x/y=w1550:dbl)
                n753 = property on="转速" class="DigNum (严格)"("Value"=w1550) -> ()  [unwired: 2 in, 2 out]
              }
              frame 60 {
                n754 = Array To Cluster(array=w1559) -> (cluster=w1565:T14)
                n755 = Unbundle By Name(w1565) -> ("Data[1]"=w1563:u8, "Data[2]"=w1562:u8)  [unwired: 1 out]
                n756 = Join Numbers(hi=w1563, lo=w1562) -> ((hi.lo)=w1564:u16)
                n757 = To Word Integer(number=w1564) -> (16bit integer=w1561:i16)
                n758 = Divide(x=w1561, y=i16 256) -> (x/y=w1558:dbl)
                n759 = property on="Iqnow" class="DigNum (严格)"("Value"=w1558) -> ()  [unwired: 2 in, 2 out]
              }
              frame 61 {
                n760 = Array To Cluster(array=w1569) -> (cluster=w1573:T14)
                n761 = Unbundle By Name(w1573) -> ("Data[1]"=w1571:u8, "Data[2]"=w1570:u8)  [unwired: 1 out]
                n762 = Join Numbers(hi=w1571, lo=w1570) -> ((hi.lo)=w1572:u16)
                n763 = To Word Integer(number=w1572) -> (16bit integer=w1568:i16)
                n764 = Divide(x=w1568, y=i16 4) -> (x/y=→"温度":dbl)
              }
              frame 64 {
                n765 = Array To Cluster(array=w1575) -> (cluster=w1580:T14)
                n766 = Unbundle By Name(w1580) -> ("Data[1]"=w1576:u8, "Data[2]"=w1577:u8)  [unwired: 1 out]
                n767 = To Unsigned Word Integer(number=w1576) -> (unsigned 16bit integer=w1583:u16)
                n768 = Rotate(1:w1583, 2:8) -> (0:w1582:u16)
                n769 = Add ("加")(x=w1582, y=w1577) -> (x+y=w1581:u16)
                n770 = Divide(x=w1581, y=u16 256) -> (x/y=→"设定位置_回":dbl)
              }
              frame 65 {
                n771 = Array To Cluster(array=w1588) -> (cluster=w1589:T14)
                n772 = Unbundle By Name(w1589) -> ("Data[1]"=w1586:u8, "Data[2]"=w1585:u8)  [unwired: 1 out]
                n773 = Join Numbers(hi=w1586, lo=w1585) -> ((hi.lo)=w1587:u16)
                n774 = To Word Integer(number=w1587) -> (16bit integer=→"设定速度_回":i16)
              }
              frame 66 {
                n775 = Array To Cluster(array=w1591) -> (cluster=w1596:T14)
                n776 = Unbundle By Name(w1596) -> ("Data[1]"=w1592:u8, "Data[2]"=w1593:u8)  [unwired: 1 out]
                n777 = To Word Integer(number=w1592) -> (16bit integer=w1599:i16)
                n778 = Rotate(1:w1599, 2:8) -> (0:w1598:i16)
                n779 = Add ("加")(x=w1598, y=w1593) -> (x+y=w1597:i16)
                n780 = Divide(x=w1597, y=u16 256) -> (x/y=→"设定电流_回":dbl)
              }
              frame 81 {
                n781 = Array To Cluster(array=w1601) -> (cluster=w1606:T14)
                n782 = Unbundle By Name(w1606) -> ("Data[1]"=w1602:u8, "Data[2]"=w1603:u8)  [unwired: 1 out]
                n783 = To Unsigned Word Integer(number=w1602) -> (unsigned 16bit integer=w1609:u16)
                n784 = Rotate(1:w1609, 2:8) -> (0:w1608:u16)
                n785 = Add ("加")(x=w1608, y=w1603) -> (x+y=w1607:u16)
                n786 = Divide(x=w1607, y=u16 256) -> (x/y=→"电流环KP_回":dbl)
              }
              frame 82 {
                n787 = Array To Cluster(array=w1611) -> (cluster=w1616:T14)
                n788 = Unbundle By Name(w1616) -> ("Data[1]"=w1612:u8, "Data[2]"=w1613:u8)  [unwired: 1 out]
                n789 = To Unsigned Word Integer(number=w1612) -> (unsigned 16bit integer=w1619:u16)
                n790 = Rotate(1:w1619, 2:8) -> (0:w1618:u16)
                n791 = Add ("加")(x=w1618, y=w1613) -> (x+y=w1617:u16)
                n792 = Divide(x=w1617, y=u16 256) -> (x/y=→"电流环KI_回":dbl)
              }
              frame 83 {
                n793 = Array To Cluster(array=w1621) -> (cluster=w1626:T14)
                n794 = Unbundle By Name(w1626) -> ("Data[1]"=w1622:u8, "Data[2]"=w1623:u8)  [unwired: 1 out]
                n795 = To Unsigned Word Integer(number=w1622) -> (unsigned 16bit integer=w1629:u16)
                n796 = Rotate(1:w1629, 2:8) -> (0:w1628:u16)
                n797 = Add ("加")(x=w1628, y=w1623) -> (x+y=w1627:u16)
                n798 = Divide(x=w1627, y=u16 256) -> (x/y=→"速度环KP_回":dbl)
              }
              frame 84 {
                n799 = Array To Cluster(array=w1631) -> (cluster=w1636:T14)
                n800 = Unbundle By Name(w1636) -> ("Data[1]"=w1632:u8, "Data[2]"=w1633:u8)  [unwired: 1 out]
                n801 = To Unsigned Word Integer(number=w1632) -> (unsigned 16bit integer=w1639:u16)
                n802 = Rotate(1:w1639, 2:8) -> (0:w1638:u16)
                n803 = Add ("加")(x=w1638, y=w1633) -> (x+y=w1637:u16)
                n804 = Divide(x=w1637, y=u16 256) -> (x/y=→"速度环KI_回":dbl)
              }
              frame 85 {
                n805 = Array To Cluster(array=w1641) -> (cluster=w1646:T14)
                n806 = Unbundle By Name(w1646) -> ("Data[1]"=w1642:u8, "Data[2]"=w1643:u8)  [unwired: 1 out]
                n807 = To Unsigned Word Integer(number=w1642) -> (unsigned 16bit integer=w1649:u16)
                n808 = Rotate(1:w1649, 2:8) -> (0:w1648:u16)
                n809 = Add ("加")(x=w1648, y=w1643) -> (x+y=w1647:u16)
                n810 = Divide(x=w1647, y=u16 8) -> (x/y=→"加速度_回":dbl)
              }
              frame 86 {
                n811 = Array To Cluster(array=w1651) -> (cluster=w1656:T14)
                n812 = Unbundle By Name(w1656) -> ("Data[1]"=w1652:u8, "Data[2]"=w1653:u8)  [unwired: 1 out]
                n813 = To Unsigned Word Integer(number=w1652) -> (unsigned 16bit integer=w1659:u16)
                n814 = Rotate(1:w1659, 2:8) -> (0:w1658:u16)
                n815 = Add ("加")(x=w1658, y=w1653) -> (x+y=w1657:u16)
                n816 = Divide(x=w1657, y=u16 8) -> (x/y=→"减速度_回":dbl)
              }
              frame 87 {
                n817 = Array To Cluster(array=w1661) -> (cluster=w1667:T14)
                n818 = Unbundle By Name(w1667) -> ("Data[1]"=w1665:u8, "Data[2]"=w1664:u8)  [unwired: 1 out]
                n819 = Join Numbers(hi=w1665, lo=w1664) -> ((hi.lo)=w1666:u16)
                n820 = To Unsigned Word Integer(number=w1666) -> (unsigned 16bit integer=w1663:u16)
                n821 = Divide(x=w1663, y=u16 8) -> (x/y=→"电流限制_回":dbl)
              }
              frame 88 {
                n822 = Array To Cluster(array=w1669) -> (cluster=w1673:T14)
                n823 = Unbundle By Name(w1673) -> ("Data[1]"=w1671:u8, "Data[2]"=w1670:u8)  [unwired: 1 out]
                n824 = Join Numbers(hi=w1671, lo=w1670) -> ((hi.lo)=w1672:u16)
                n825 = To Unsigned Word Integer(number=w1672) -> (unsigned 16bit integer=→"速度限制_回":u16)
              }
              frame 90 {
                n826 = Array To Cluster(array=w1678) -> (cluster=w1679:T14)
                n827 = Unbundle By Name(w1679) -> ("Data[1]"=w1676:u8, "Data[2]"=w1675:u8)  [unwired: 1 out]
                n828 = Join Numbers(hi=w1676, lo=w1675) -> ((hi.lo)=w1677:u16)
                n829 = To Unsigned Word Integer(number=w1677) -> (unsigned 16bit integer=→"AI_K0_回":u16)
              }
              frame 91 {
                n830 = Array To Cluster(array=w1681) -> (cluster=w1685:T14)
                n831 = Unbundle By Name(w1685) -> ("Data[1]"=w1683:u8, "Data[2]"=w1682:u8)  [unwired: 1 out]
                n832 = Join Numbers(hi=w1683, lo=w1682) -> ((hi.lo)=w1684:u16)
                n833 = To Unsigned Word Integer(number=w1684) -> (unsigned 16bit integer=→"BI_K0_回":u16)
              }
              frame 92 {
                n834 = Array To Cluster(array=w1687) -> (cluster=w1691:T14)
                n835 = Unbundle By Name(w1691) -> ("Data[1]"=w1689:u8, "Data[2]"=w1688:u8)  [unwired: 1 out]
                n836 = Join Numbers(hi=w1689, lo=w1688) -> ((hi.lo)=w1690:u16)
                n837 = To Unsigned Word Integer(number=w1690) -> (unsigned 16bit integer=→"CI_K0_回":u16)
              }
              frame 93 {
                n838 = Array To Cluster(array=w1695) -> (cluster=w1699:T14)
                n839 = Unbundle By Name(w1699) -> ("Data[1]"=w1697:u8, "Data[2]"=w1696:u8)  [unwired: 1 out]
                n840 = Join Numbers(hi=w1697, lo=w1696) -> ((hi.lo)=w1698:u16)
                n841 = To Unsigned Word Integer(number=w1698) -> (unsigned 16bit integer=w1694:u16)
                n842 = Divide(x=w1694, y=u16 8) -> (x/y=→"对准角_回":dbl)
              }
              frame 94 {
                n843 = Array To Cluster(array=w1701) -> (cluster=w1702:cluster{"Data[0]":u8, "Data[1]":u8})
                n844 = Unbundle By Name(w1702) -> ("Data[1]"=→"极对数_回":u8)  [unwired: 1 out]
              }
              frame 95 {
                n845 = Array To Cluster(array=w1704) -> (cluster=w1708:T14)
                n846 = Unbundle By Name(w1708) -> ("Data[1]"=w1706:u8, "Data[2]"=w1705:u8)  [unwired: 1 out]
                n847 = Join Numbers(hi=w1706, lo=w1705) -> ((hi.lo)=w1707:u16)
                n848 = To Unsigned Word Integer(number=w1707) -> (unsigned 16bit integer=→"编码器线数_回":u16)
              }
            }
            n849 = case shown="真" w1299 {
              tunnel: w1298 -> [_ w1309]
              tunnel: w1297 -> [_ w1307]
              frame False {
              }
              frame True {
                n850 = Array Size(array=w1307) -> (size(s)=w1308:i32)
                n851 = Open/Create/Replace File(file path (use dialog)=w1309, operation (0:open)=T11."open or create") -> (refnum out=w1317:refnum<file>, error out=w1306:errorcluster)  [unwired: 4 in, 1 out]
                n852 = for {
                  N: w1308 -> [_]
                  shift-right: [w1325] -> w1314
                  shift-left: "" -> [w1322]
                  tunnel: w1307 -> [w1320]
                  i -> [w1321]
                  # "浮点文本存储"
                  # "2-14"
                  n853 = Index Array(array=w1320, index=w1321) -> (element=w1319:dbl)
                  n854 = Number To Fractional String(number=w1319) -> (F-format string=w1324:string)  [unwired: 3 in]
                  n855 = Concatenate Strings(w1322, w1324, "\t") -> (w1325:string)
                }
                n856 = Set File Position(refnum=w1317, from (0:start)=u16 1, error in=w1306) -> (refnum out=w1316:refnum<file>, error out=w1305:errorcluster)  [unwired: 1 in]
                n857 = Concatenate Strings(w1314, "\r") -> (w1312:string)
                n858 = Write to Text File(file (use dialog)=w1316, text=w1312, error in=w1305) -> (refnum out=w1315:refnum<file>, error out=w1304:errorcluster)  [unwired: 1 in, 1 out]
                n859 = Close File(refnum=w1315, error in=w1304) -> (error out=w1303:errorcluster)  [unwired: 1 out]
                n860 = call <vilib>:"Clear Errors.vi"("error in (no error)"=w1303) -> ()  [unwired: 6 in, 1 out]
              }
            }
          }
        }
      }
      frame True {
      }
    }
  }
  n861 = while "接收线程" {
    tunnel: w9 -> [w1712]
    shift-right: [w1710] -> _
    shift-left: u32 0 ("RecvCnt") -> [w1711]
    stop <- "RcvEnable" continue-if-true
    n862 = local read "Open"() -> (w1713:bool)
    n863 = case shown="真" w1713 {
      tunnel: w1712 -> [_ w1720]
      tunnel: w1711 -> [w1715 w1719]
      tunnel: [w1715 w1718] -> w1710
      frame False {
        # "CAN未打开，延时50ms"
        n864 = Wait (ms)(milliseconds to wait=u32 50 ("等待时间（毫秒）")) -> ()  [unwired: 1 out]
      }
      frame True {
        n865 = local read "DevType"() -> (w1724:T5)
        n866 = local read "Channel"() -> (w1717:T4)
        n867 = call "VCI_Receive.vi"("CANIndex"=w1717, "DevIndex"=u32 0, "DevType"=w1724) -> ("Recieve"=w1721:T6[])  [unwired: 3 in, 5 out]
        n868 = Empty Array?(array=w1721) -> (empty?=w1722:bool)
        n869 = case shown="假" w1722 {
          tunnel: w1720 -> [w1731 _]
          tunnel: w1721 -> [w1726 _]
          tunnel: [w1730 _] -> _
          tunnel: w1719 -> [w1728 w1743]
          tunnel: [w1727 w1743] -> w1718
          tunnel: w1717 -> [w1729 _]
          frame False {
            n870 = Array Size(array=w1726) -> (size(s)=w1725:i32)
            n871 = for {
              N: w1725 -> [_]
              tunnel: w1731 -> [w1742]
              tunnel: [w1740] -> w1730 mode=indexing
              tunnel: w1726 -> [w1735]
              tunnel: w1729 -> [w1739]
              shift-right: [w1736] -> w1727
              shift-left: w1728 -> [w1737]
              i -> [w1733]
              n872 = Array Subset(array=w1735, index=w1733, length=1) -> (w1734:T6[])
              n873 = Increment(x=w1737) -> (x+1=w1736:u32)
              n874 = call "Demo_MakeDispBuff.vi"("Channel"=w1739, "Type"=enum16{"接收", "发送"}."接收", "OBJs"=w1734) -> ("Buffer"=w1741:T7)
              n875 = Enqueue Element(queue=w1742, element=w1741) -> (error out=w1740:errorcluster)  [unwired: 1 in, 3 out]
            }
            "RecvCnt" <- w1727
          }
          frame True {
          }
        }
      }
    }
  }
  n876 = control-ref of="本应用程序"() -> (w6:refnum<vi>)
  n877 = invoke class="VI" method="FP.Close"(error in=w4) -> (error out=w3:errorcluster)  [unwired: 2 in, 2 out]
  n878 = property class="App"(reference=w6) -> ("App.Kind"=w5:T16)  [unwired: 1 in, 2 out]
  n879 = case shown="\"Development System\"" w5 {
    tunnel: w3 -> [_ _]
    frame "invalid app kind", Default {
      n880 = Quit LabVIEW() -> ()  [unwired: 1 out]
    }
    frame "Development System" {
    }
  }
